vi "mec.vi"() -> ()   [LabVIEW 2016]
uses:
  <instrlib>/ZaberTSeries/Public/Utility/Request.ctl
  <instrlib>/Lake Shore 350/Public/Data/Sensor Data (Single Reading).vi
  <vilib>/Utility/file.llb/Write Delimited Spreadsheet (string).vi
  <vilib>/Utility/file.llb/Write Delimited Spreadsheet (DBL).vi
  <instrlib>/Lake Shore 372/Lake Shore 372.lvlib
  <instrlib>/Lake Shore 350/Lake Shore 350.lvlib
  <instrlib>/Lake Shore Cryotronics 370/Lake Shore Cryotronics 370.lvlib
  <instrlib>/ZaberTSeries/ZaberTSeries.lvlib
panel:
  in  "Stop":bool=TRUE
  out "current time":timestamp format="%<%I:%M:%S %p>T"
  in  "Tab Control":T1(tab)=enum."Ramp Config"
  out "Reading 370":bool
  out "Arduino OK":bool
  out "PT1":waveform(dbl)(graph)
  out "stopping":bool=TRUE
  out "FAA RO600":dbl caption="FAA (K)" min=0.0 max=63200000.0 step=1e-05 format="%_4f"
  out "Sample RuOx":dbl caption="Device (K)" min=0.0 max=63200000.0 step=1e-05 format="%_3f"
  out "Magnet Current (A)":dbl format="%.3f"
  out "77K Diode":dbl format="%_4f"
  out "4K Diode":dbl format="%_4f"
  out "Magnetic Field (kG)":dbl min=-601000.0 max=601000.0 step=0.0001 format="%_3f"
  in  "Auto-Ramp":bool
  in  "ramp start time":timestamp
  out "Ramp Status":string="Shutting down"
  out "Ramp State":u16(ring)=6 items=["Ramp Up", "Soak (hold)", "Ramp Down", "Ramp up to Setpoint", "Closed Loop Feedback", "Ramp down from Setpoint", "Magnet off"]
  out "Magnet Current":waveform(dbl)[](graph)
  out "Device T":waveform(dbl)(graph)
  out "Sample RuOx R":dbl caption="Device R (Ohms)" min=0.0 max=63200000.0 step=1e-05 format="%_3f"
  out "FAA RO600 R":dbl caption="FAA R (Ohms)" min=0.0 max=63200000.0 step=1e-05 format="%_4f"
  out "Magnet RTD":dbl caption="Magnet (K)" format="%.2f"
  out "GGG RO600":dbl caption="GGG (K)" format="%_4f"
  out "GGG RO600 R":dbl caption="GGG R (Ohms)" format="%_4f"
  out "Magnet RTD R":dbl caption="Magnet R (Ohms)" format="%.2f"
  out "PT2":waveform(dbl)(graph)
  in  "magnet control resistance ohms":dbl=20.0
  in  "Calculate Autoramp Time":bool
  in  "End of Ramp Temp Control":bool=TRUE
  in  "soak time (minutes)":dbl=50.0
  out "cycle time (min)":dbl format="%#_3g"
  out "Ramp down step size (mA)":dbl=1.0
  in  "setpoint (K)":dbl=0.09
  in  "Manual temp control":bool
  in  "ls350":refnum<visa-resource-name>="350"
  in  "ls370":refnum<visa-resource-name>="370"
  out "Ramp up step size (%)":dbl=0.02
  out "max magnet value(%)":dbl=10.0
  in  "read lakeshore sensors":bool=TRUE
  in  "Record Temps":bool=TRUE
  in  "Timeout (ms)":i32=2000
  out "Ramp up step size (mA)":dbl=1.0
  in  "Max current (A)":dbl=9.4
  in  "thermo data path":path=path "C:/data/temperature_log/mec"
  in  "Field constant (kG/A)":dbl=4.566 min=0.001 max=10.0 step=1e-05 format="%.3f"
  out "Ramp down step size (%)":dbl=0.02
  out "ramp up time (min)":dbl=60.0
  out "ramp down time (min)":dbl=60.0
  out "ramp down start time":timestamp
  in  "Ramp up rate (mA/s)":dbl=5.0
  in  "Ramp down rate (mA/s)":dbl=5.0
  in  "Heat Switch":bool
  in  "Ramp Magnet Up":bool
  in  "Ramp Magnet Down":bool
  in  "control channel":string="1"
  out "counter":dbl
  in  "delay after ramp down (min)":dbl=20.0
  out "counter 2":dbl
  out "ramp finish time":timestamp
  out "lakeshore output %":dbl format="%.3f"
  out "Heater Range Set":u16(ring) items=["Off", "31.6 uA", "100 uA", "316 uA", "1.00 mA", "3.16 mA", "10.0 mA", "31.6 mA", "100 mA"]
  out "Heater Range Actual":u16(ring) items=["Off", "31.6 uA", "100 uA", "316 uA", "1.00 mA", "3.16 mA", "10.0 mA", "31.6 mA", "100 mA"]
  out "Magnet resistance ohms":dbl=1.0
  out "Heater Range OK":bool
  out "heater Setpoint":dbl min=0.0 max=100000000.0 step=1e-06 format="%.5f"
  out "lakeshore output current mA":dbl
  out "kepco input voltage (V)":dbl
  out "kepco output voltage (V)":dbl
  out "Magnet Current (A) 2":dbl format="%.3f"
  in  "magnet ramp resistance ohms":dbl=0.1005
  in  "Update PID Values":bool
  in  "Warmup Heater":bool=TRUE
  in  "Channel (1)":u16(ring)=1 items=["1"=1, "2"=2, "3"=3, "4"=4, "5"=5, "6"=6, "7"=7, "8"=8, "9"=9, "10"=10, "11"=11, "12"=12, "13"=13, "14"=14, "15"=15, "16"=16, "A (Control Input)"=17]
  in  "Excitation Range (5: 200 uV / 100 pA)":u16(ring)=5 items=["2.00 uV / 1.00 pA"=1, "6.32 uV / 3.16 pA"=2, "20.0 uV / 10.0 pA"=3, "63.2 uV / 31.6 pA"=4, "200 uV / 100 pA"=5, "632 uV / 316 pA"=6, "2.00 mV / 1.00 nA"=7, "6.32 mV / 3.16 nA"=8, "20.0 mV / 10.0 nA"=9, "63.2 mV / 31.6 nA"=10, "200 mV / 100 nA"=11, "632 mV / 316 nA"=12, "1.00 uA"=13, "3.16 uA"=14, "10.0 uA"=15, "31.6 uA"=16, "100 uA"=17, "316 uA"=18, "1.00 mA"=19, "3.16 mA"=20, "10.0 mA"=21, "31.6 mA"=22]
  in  "Autorange (0: Autorange off)":u16(ring) items=["Autorange off", "Autorange Current", "ROX 102B Autorange"]
  in  "Excitation  (T: On)":bool=TRUE
  in  "Excitation Mode (0: Voltage)":u16(ring) items=["Voltage", "Current"]
  in  "Resistance Range (17: 200 kOhm)":u16(ring)=17 items=["2.00 mOhm"=1, "6.32 mOhm"=2, "20.0 mOhm"=3, "63.2 mOhm"=4, "200 mOhm"=5, "632 mOhm"=6, "2.00 Ohm"=7, "6.32 Ohm"=8, "20.0 Ohm"=9, "63.2 Ohm"=10, "200 Ohm"=11, "632 Ohm"=12, "2.00 kOhm"=13, "6.32 kOhm"=14, "20.0 kOhm"=15, "63.2 kOhm"=16, "200 kOhm"=17, "632 kOhm"=18, "2.00 MOhm"=19, "6.32 MOhm"=20, "20.0 MOhm"=21, "63.2 MOhm"=22]
  in  "Gain(P)":dbl=1.1 min=0.001 max=1000.0 step=0.001 format="%.3f"
  in  "Reset(I)":dbl=30.0 min=0.0 max=10000.0 step=1.0
  in  "Rate(D)":dbl min=0.0 max=2500.0 step=1.0
  in  "Mode (0:Off)":u16(ring)=3 items=["Off", "Closed Loop PID", "Zone", "Open Loop"]
  in  "Heater Output (1:1)":u16(ring)=1 items=["1"=1, "2"=2]
  in  "Input (0:None)":u16(ring)=6 items=["None", "A", "B", "C", "D", "D2", "D3", "D4", "D5"]
  in  "Max Current (0:User Specified)":u16(ring) items=["User Specified", "0.707 A", "1.0 A", "1.141 A", "2.0 A"]
  in  "Heater Out Display (1:Current)":u16(ring)=1 items=["Current"=1, "Power"=2]
  in  "Max User Current (2.000)":dbl=0.1 format="%.3f"
  in  "Heater Resistance (1:25 Ohms)":u16(ring)=2 items=["25 Ohms"=1, "50 Ohms"=2]
  in  "heater output":u16(ring)=1 items=["1"=1, "2"=2, "3"=3, "4"=4]
  in  "warmup heater Range":u16(ring) items=["Off", "Range 1 (On)", "Range 2", "Range 3", "Range 4", "Range 5"]
  in  "warmup heater output %":dbl=62.0 format="%.2f"
  in  "Knob":i8(knob) scale=0.0..2.0
  in  "auto-read HEMT voltages":bool=TRUE
  in  "Read ADC current":bool=TRUE
  in  "query adc magnet current once":bool
  in  "MUX relays":bool
  in  "Query all HEMT voltages once":bool
  out "HEMT biases":dbl[][](array[numeric])
  out "ADC0 outputs":dbl[][](array[numeric])
  out "adc magnet current (A)":dbl
  in  "Arduino":refnum<visa-resource-name>="COM6"
  out "flow meter":dbl
  out "hemt v counter":i32
  out "element":string
  out "last record time":dbl
  in  "HEMT data path":path=path "C:/data/temperature_log/mec"
  out "error out":errorcluster
  out "Flow Meter":waveform(dbl)(graph)
  out "FAA T":waveform(dbl)(graph)={"t0"=timestamp(3512160360.4800687 s since 1904-01-01), "dt"=0.0, "Y"=[0.0]}
  out "GGG T":waveform(dbl)(graph)={"t0"=timestamp(3512160360.4800687 s since 1904-01-01), "dt"=0.0, "Y"=[0.0]}
  out "magnet RTD R":waveform(dbl)(graph)={"t0"=timestamp(3512160360.4800687 s since 1904-01-01), "dt"=0.0, "Y"=[0.0]}
  in  "initialize":bool
  # "MEC!"
  # "ADR CONTROL"
  # "Manual ADR CONTROL"
  # "How often to measure temps?\nDon't change this during ramps."
  # "OPEN"
  # "CLOSED"
  # "Ramp Parameters"
  # "\"A\" for Darkness \n\"1\" for MEC"
  # "Lakeshore 370"
  # "Warmup Heater (LS350)"
  # "Temp Control Parameters\nLS370"
  # "ON"
  # "OFF"
  # "ARCONS used 1.1, 60, and 15 for PID"
  # "A1"
  # "A2"
  # "A3"
  # "OFF"
  # "ON"
  # "A4"
  # "A5"
  # "B1"
  # "OPEN"
  # "CLOSED"
  # "B2"
  # "last HEMT voltage polled:"
  # "B3"
  # "B4"
  # "B5"
  # "Vd (mV)"
  # "Id (mAx100)"
  # "Vg (mV)"
  # "magnet \ncurrent"
  # "flow \nmeter"
  # "OFF"
  # "ON"
  # "Thermometers\n\nFrom DARKNESS\nUse ~ 20 uV or ~20 nA excitation for FAA and device thermometers. \nHPD recommendations (these are conservative. Scientific instruments used excitations that were 10 to 100 times higher)\nT(K)                            excitation (nA)\n.175 to 4.2                  10\n.1 to .175                    3\n<.1                              0.1\n\nDiodes get 10 uA excitation. \n\n\nKepco Front Panel\nVoltage Control = OFF\nCurrent Control = OFF\nMode = Voltage\n\nSample Heater Output from LS372 connects to Voltage Programming Input on Kepco. Red terminal on front of Kepco should\nget a voltage <0, Red magnet wire goes to OUT on back of Kepco, Blue wire goes to COM on back of Kepco."
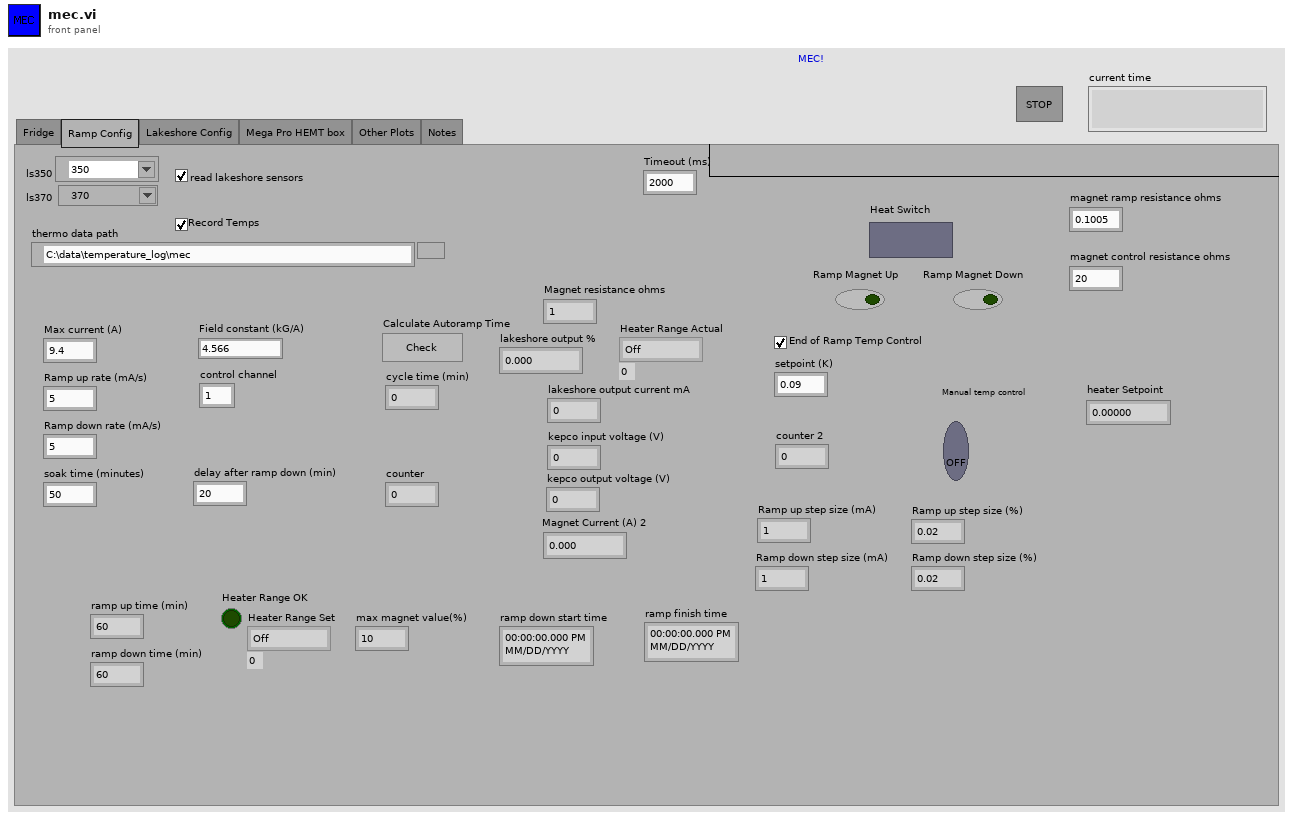
[diagram p1: front panel]
types:
  T1 = enum32{"Fridge", "Ramp Config", "Lakeshore Config", "Mega Pro HEMT box", "Other Plots", "Notes"}
  T2 = typedef "ZaberTSeries.lvlib/Request.ctl" = cluster{"Device Number":u8, "Command":u8, "Data":i32, "Response Count":i32}
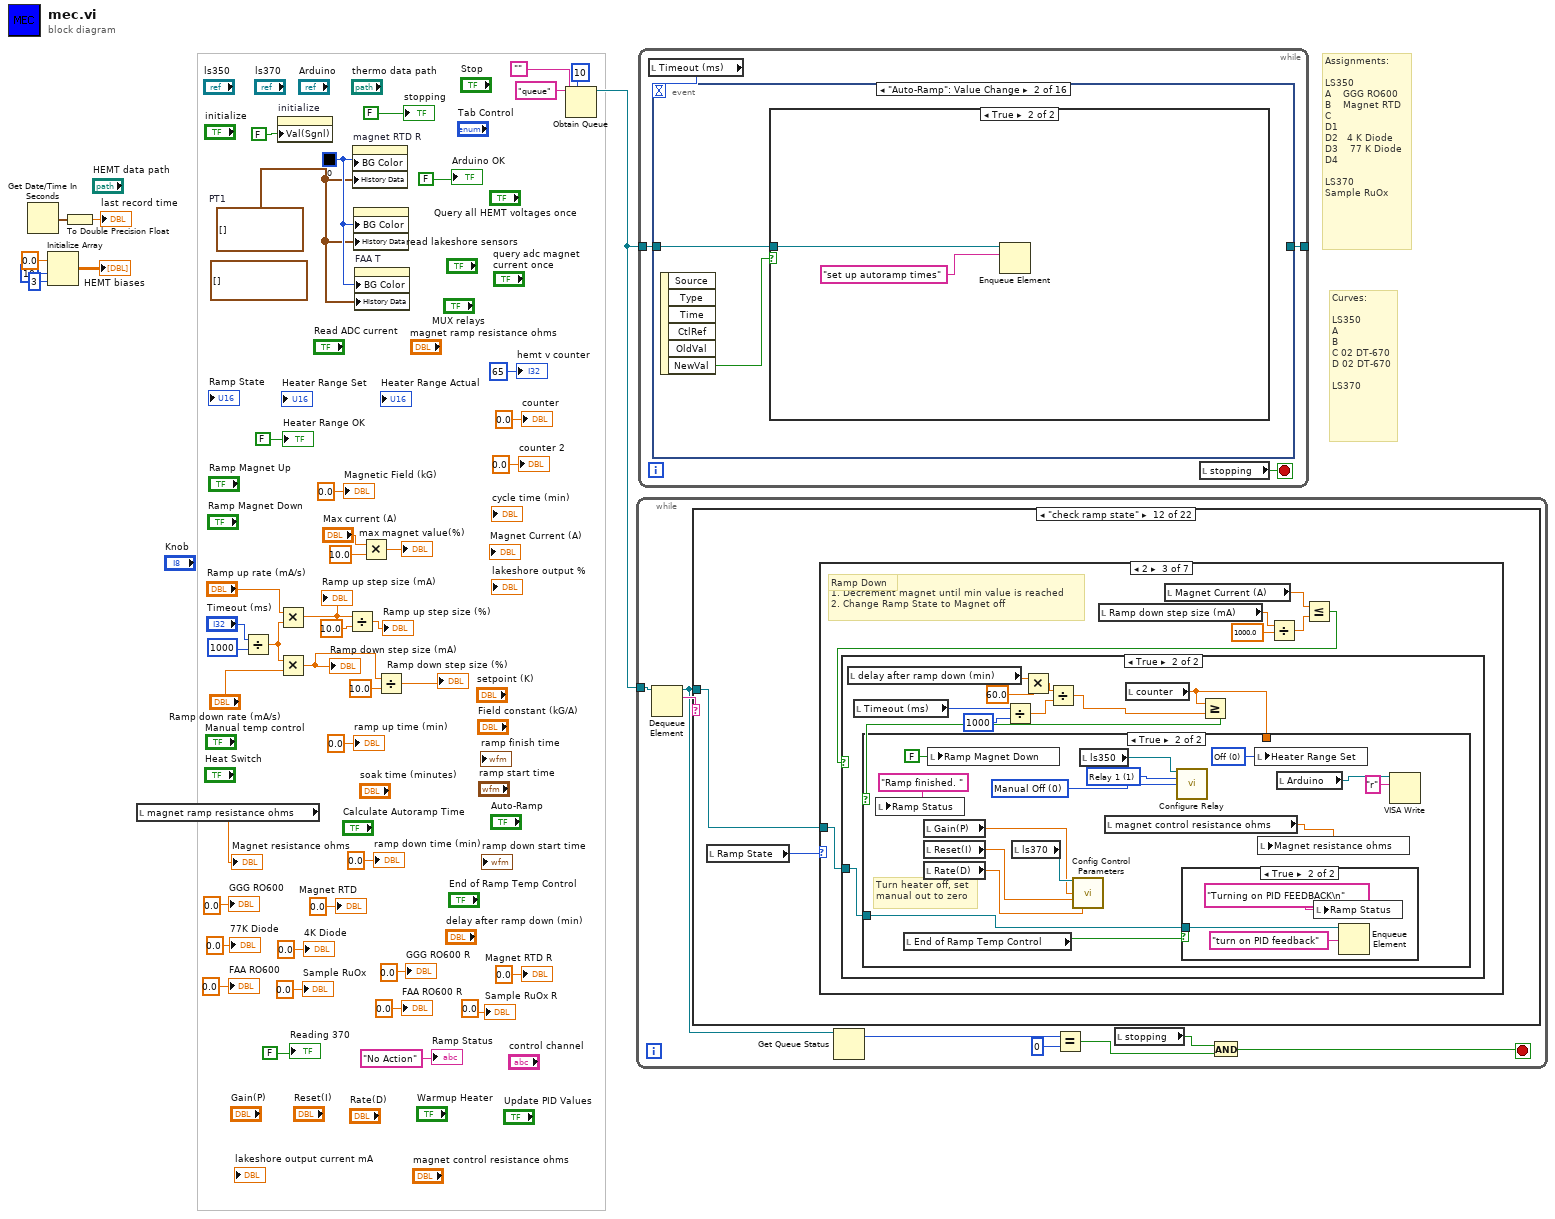
[diagram p0: block diagram]
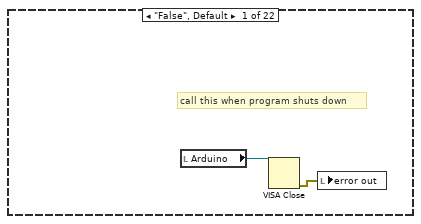
[diagram p2: hidden frame]
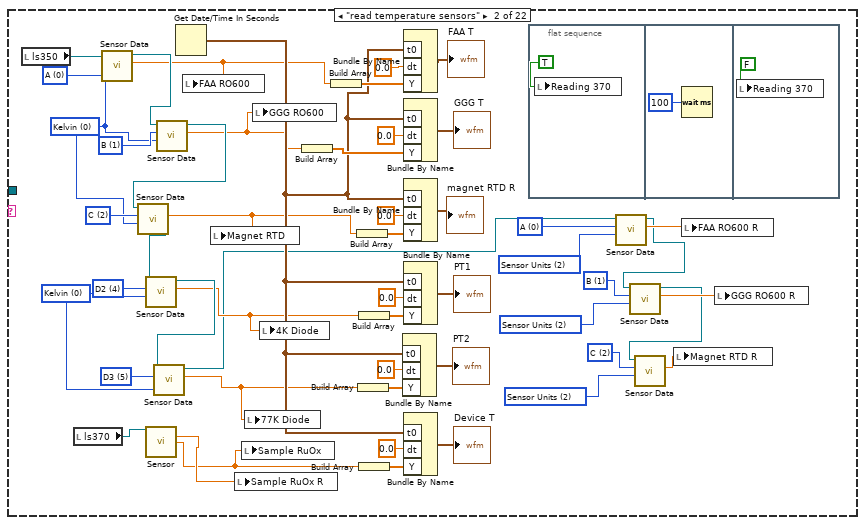
[diagram p3: hidden frame]
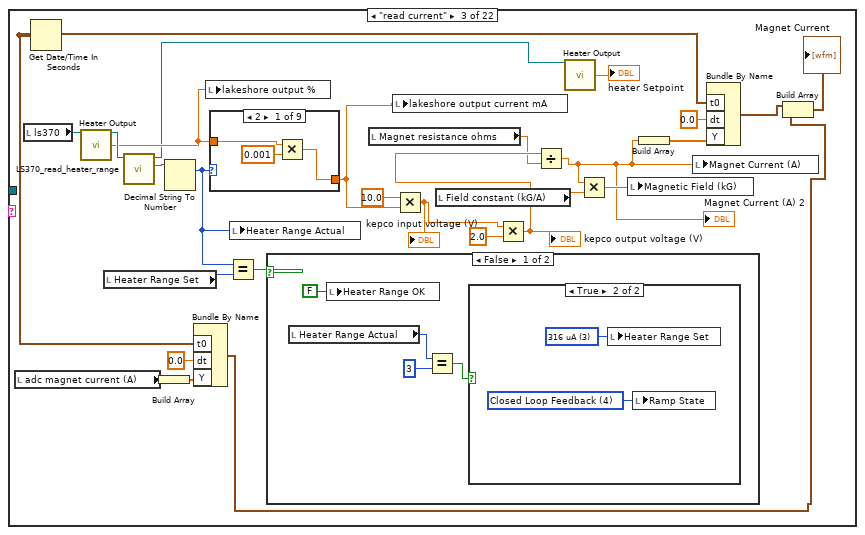
[diagram p4: hidden frame]
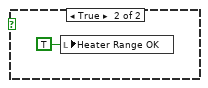
[diagram p6: hidden frame]
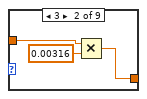
[diagram p7: hidden frame]
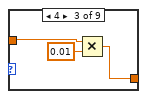
[diagram p8: hidden frame]
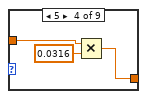
[diagram p9: hidden frame]
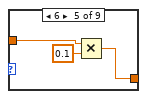
[diagram p10: hidden frame]
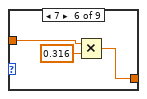
[diagram p11: hidden frame]
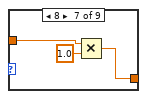
[diagram p12: hidden frame]
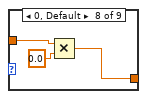
[diagram p13: hidden frame]
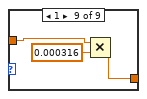
[diagram p14: hidden frame]
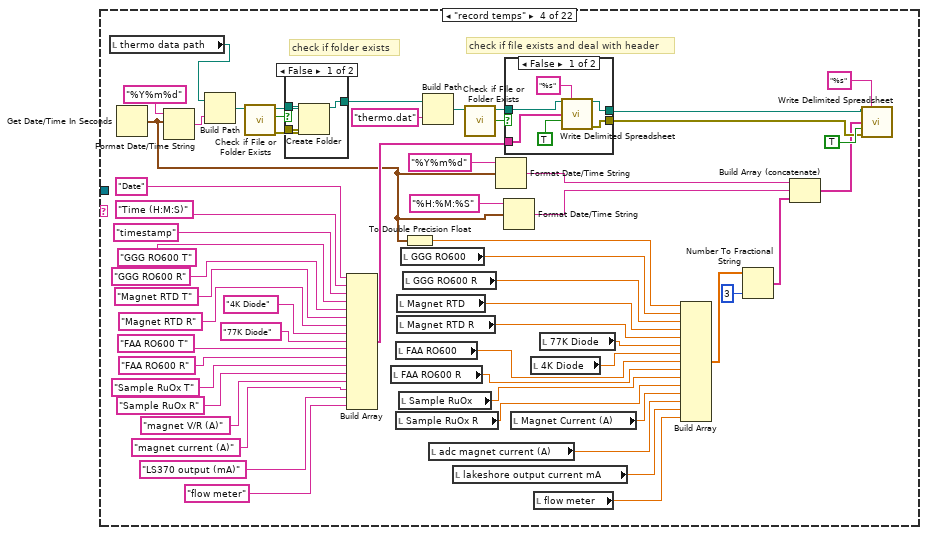
[diagram p15: hidden frame]
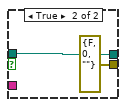
[diagram p16: hidden frame]
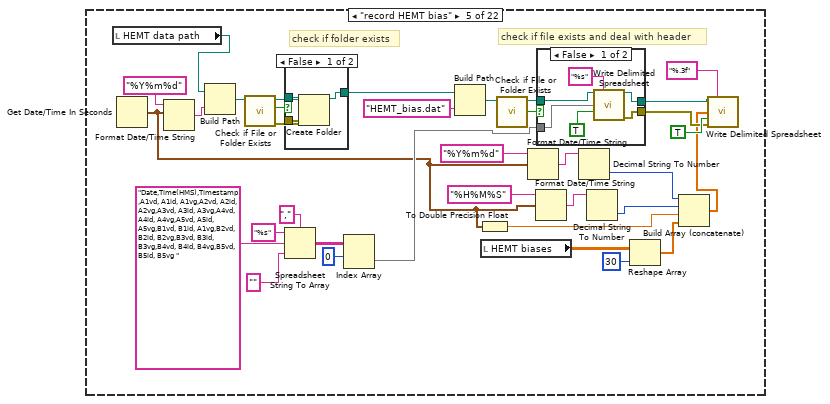
[diagram p18: hidden frame]
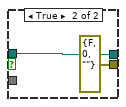
[diagram p19: hidden frame]
diagram:
  (unwired) waveform(dbl)[][] [] ("History Data")
  w9 = waveform(dbl)[] [] ("History Data")
  w39 = u32 0
  # "Curves:\n\nLS350\nA\nB\nC 02 DT-670\nD 02 DT-670\n\nLS370"
  # "Assignments:\n\nLS350\nA    GGG RO600 \nB    Magnet RTD\nC\nD1\nD2   4 K Diode\nD3    77 K Diode\nD4\n\nLS370\nSample RuOx"
  n1 = Get Date/Time In Seconds() -> (seconds since 1Jan1904=w6:timestamp)
  n2 = Initialize Array(0.0 ("element"), 10 ("dimension size"), 3 ("dimension size")) -> (→"HEMT biases":dbl[][])
  n3 = To Double Precision Float(number=w6) -> (double precision float=→"last record time":dbl)
  n4 = local read "magnet ramp resistance ohms"() -> (→"Magnet resistance ohms":dbl)
  n5 = Divide(x="Timeout (ms)", y=1000) -> (x/y=w19:dbl)
  n6 = property on="initialize" class="Bool (strict)"("Val(Sgnl)"=FALSE ("Boolean")) -> ()  [unwired: 2 in, 2 out]
  n7 = Multiply(x="Ramp up rate (mA/s)", y=w19) -> (x*y=w16:dbl)
  "Ramp up step size (mA)" <- w16
  n8 = Multiply(x=w19, y="Ramp down rate (mA/s)") -> (x*y=w17:dbl)
  "Ramp down step size (mA)" <- w17
  n9 = Divide(x=w16, y=10.0) -> (x/y=→"Ramp up step size (%)":dbl)
  n10 = property on="magnet RTD R" class="WFChart (strict)"("BG Color"=w39, "History Data"=w9) -> ()  [unwired: 2 in, 2 out]
  n11 = property on="PT1" class="WFChart (strict)"("BG Color"=w39, "History Data"=w9) -> ()  [unwired: 2 in, 2 out]
  n12 = property on="FAA T" class="WFChart (strict)"("BG Color"=w39, "History Data"=w9) -> ()  [unwired: 2 in, 2 out]
  n13 = Multiply(x="Max current (A)", y=10.0) -> (x*y=→"max magnet value(%)":dbl)
  n14 = Divide(x=w17, y=10.0) -> (x/y=→"Ramp down step size (%)":dbl)
  n15 = Obtain Queue(max queue size (-1, unlimited)=10, name (unnamed)="queue", element data type="") -> (queue out=w47:refnum<queue>)  [unwired: 2 in, 2 out]
  n16 = while {
    tunnel: w47 -> [w57]
    stop <- w51 stop-if-true
    n17 = Dequeue Element(queue=w57) -> (queue out=w50:refnum<queue>, element=w56:string)  [unwired: 2 in, 2 out]
    n18 = case shown="\"check ramp state\"" w56 {
      tunnel: w50 -> [_ _ _ _ _ _ _ _ _ _ _ w489 _ _ _ _ _ _ _ _ _ _]
      frame "False", Default {
        # "call this when program shuts down"
        n19 = local read "Arduino"() -> (w59:refnum<visa-resource-name>)
        n20 = VISA Close(VISA resource name=w59) -> (error out=w58:errorcluster)  [unwired: 1 in]
        n21 = local write "error out"(w58) -> ()
      }
      frame "read temperature sensors" {
        w61 = u16 2 items=["Kelvin", "Celsius", "Sensor Units"] ("Data Source (0:Kelvin)")
        w63 = u16 2 items=["A", "B", "C", "D", "D2", "D3", "D4", "D5"] ("Input (0:A)")
        w67 = u16 2 items=["Kelvin", "Celsius", "Sensor Units"] ("Data Source (0:Kelvin)")
        w65 = u16 1 items=["A", "B", "C", "D", "D2", "D3", "D4", "D5"] ("Input (0:A)")
        w70 = u16 2 items=["Kelvin", "Celsius", "Sensor Units"] ("Data Source (0:Kelvin)")
        w71 = u16 0 items=["A", "B", "C", "D", "D2", "D3", "D4", "D5"] ("Input (0:A)")
        w94 = u16 5 items=["A", "B", "C", "D", "D2", "D3", "D4", "D5"] ("Input (0:A)")
        w92 = u16 0 items=["Kelvin", "Celsius", "Sensor Units"] ("Data Source (0:Kelvin)")
        w95 = u16 4 items=["A", "B", "C", "D", "D2", "D3", "D4", "D5"] ("Input (0:A)")
        w99 = u16 2 items=["A", "B", "C", "D", "D2", "D3", "D4", "D5"] ("Input (0:A)")
        w97 = u16 0 items=["Kelvin", "Celsius", "Sensor Units"] ("Data Source (0:Kelvin)")
        w100 = u16 1 items=["A", "B", "C", "D", "D2", "D3", "D4", "D5"] ("Input (0:A)")
        w104 = u16 0 items=["A", "B", "C", "D", "D2", "D3", "D4", "D5"] ("Input (0:A)")
        n22 = local read "ls350"() -> (w105:refnum<visa-resource-name>)
        n23 = local read "ls370"() -> (w83:refnum<visa-resource-name>)
        n24 = call-poly <instrlib>:"Sensor Data.vi"("Data Source (0:Kelvin)"=w97, "Input (0:A)"=w104, "VISA resource name"=w105) -> ("Sensor Data"=w78:dbl, "VISA resource name out"=w101:refnum<visa-resource-name>)  [unwired: 6 in, 1 out]
        n25 = call <instrlib>:"Sensor.vi"("VISA resource name"=w83) -> ("Resistance Reading"=w74:dbl, "Kelvin Reading"=w73:dbl)  [unwired: 10 in, 3 out]
        n26 = call-poly <instrlib>:"Sensor Data.vi"("Data Source (0:Kelvin)"=w97, "Input (0:A)"=w100, "VISA resource name"=w101) -> ("Sensor Data"=w69:dbl, "VISA resource name out"=w98:refnum<visa-resource-name>)  [unwired: 6 in, 1 out]
        n27 = call-poly <instrlib>:"Sensor Data.vi"("Data Source (0:Kelvin)"=w97, "Input (0:A)"=w99, "VISA resource name"=w98) -> ("Sensor Data"=w77:dbl, "VISA resource name out"=w96:refnum<visa-resource-name>)  [unwired: 6 in, 1 out]
        n28 = call-poly <instrlib>:"Sensor Data.vi"("Data Source (0:Kelvin)"=w92, "Input (0:A)"=w95, "VISA resource name"=w96) -> ("Sensor Data"=w75:dbl, "VISA resource name out"=w93:refnum<visa-resource-name>)  [unwired: 6 in, 1 out]
        n29 = call-poly <instrlib>:"Sensor Data.vi"("Data Source (0:Kelvin)"=w92, "Input (0:A)"=w94, "VISA resource name"=w93) -> ("Sensor Data"=w76:dbl, "VISA resource name out"=w72:refnum<visa-resource-name>)  [unwired: 6 in, 1 out]
        n30 = Get Date/Time In Seconds() -> (seconds since 1Jan1904=w79:timestamp)
        n31 = local write "FAA RO600"(w78) -> ()
        n32 = local write "Magnet RTD"(w77) -> ()
        n33 = local write "Sample RuOx R"(w74) -> ()
        n34 = local write "Sample RuOx"(w73) -> ()
        n35 = local write "77K Diode"(w76) -> ()
        n36 = local write "GGG RO600"(w69) -> ()
        n37 = local write "4K Diode"(w75) -> ()
        n38 = Build Array(w69) -> (w90:dbl[])
        n39 = Build Array(w78) -> (w102:dbl[])
        n40 = Build Array(w77) -> (w89:dbl[])
        n41 = Build Array(w76) -> (w84:dbl[])
        n42 = Build Array(w75) -> (w87:dbl[])
        n43 = Build Array(w73) -> (w82:dbl[])
        n44 = Bundle By Name("t0"=w79, "dt"=0.0, "Y"=w84) -> (→"PT2":waveform(dbl))  [unwired: 1 in]
        n45 = Bundle By Name("t0"=w79, "dt"=0.0, "Y"=w102) -> (→"FAA T":waveform(dbl))  [unwired: 1 in]
        n46 = Bundle By Name("t0"=w79, "dt"=0.0, "Y"=w90) -> (→"GGG T":waveform(dbl))  [unwired: 1 in]
        n47 = Bundle By Name("t0"=w79, "dt"=0.0, "Y"=w89) -> (→"magnet RTD R":waveform(dbl))  [unwired: 1 in]
        n48 = Bundle By Name("t0"=w79, "dt"=0.0, "Y"=w87) -> (→"PT1":waveform(dbl))  [unwired: 1 in]
        n49 = Bundle By Name("t0"=w79, "dt"=0.0, "Y"=w82) -> (→"Device T":waveform(dbl))  [unwired: 1 in]
        n50 = flat-sequence {
          frame #0 {
            n51 = local write "Reading 370"(TRUE ("Reading 370")) -> ()
          }
          frame #1 {
            n52 = Wait (ms)(milliseconds to wait=u32 100) -> ()  [unwired: 1 out]
          }
          frame #2 {
            n53 = local write "Reading 370"(FALSE ("Reading 370")) -> ()
          }
        }
        n54 = call-poly <instrlib>:"Sensor Data.vi"("Data Source (0:Kelvin)"=w70, "Input (0:A)"=w71, "VISA resource name"=w72) -> ("Sensor Data"=w68:dbl, "VISA resource name out"=w64:refnum<visa-resource-name>)  [unwired: 6 in, 1 out]
        n55 = call-poly <instrlib>:"Sensor Data.vi"("Data Source (0:Kelvin)"=w67, "Input (0:A)"=w65, "VISA resource name"=w64) -> ("Sensor Data"=w66:dbl, "VISA resource name out"=w60:refnum<visa-resource-name>)  [unwired: 6 in, 1 out]
        n56 = call-poly <instrlib>:"Sensor Data.vi"("Data Source (0:Kelvin)"=w61, "Input (0:A)"=w63, "VISA resource name"=w60) -> ("Sensor Data"=w62:dbl)  [unwired: 6 in, 2 out]
        n57 = local write "Magnet RTD R"(w62) -> ()
        n58 = local write "FAA RO600 R"(w68) -> ()
        n59 = local write "GGG RO600 R"(w66) -> ()
      }
      frame "read current" {
        n60 = local read "adc magnet current (A)"() -> (w119:dbl)
        n61 = local read "ls370"() -> (w138:refnum<visa-resource-name>)
        n62 = Get Date/Time In Seconds() -> (seconds since 1Jan1904=w115:timestamp)
        n63 = call <instrlib>:"Heater Output.vi"("VISA resource name"=w138) -> ("VISA resource name out"=w137:refnum<visa-resource-name>, "Heater Output"=w132:dbl)  [unwired: 12 in, 1 out]
        n64 = local read "Heater Range Set"() -> (w134:u16)
        n65 = call "LS370_read_heater_range.vi"("VISA resource name"=w137) -> ("heater range"=w136:string, "VISA resource name out"=w129:refnum<visa-resource-name>)  [unwired: 9 in]
        n66 = Build Array(w119) -> (w120:dbl[])
        n67 = Decimal String To Number(string=w136) -> (number=w135:i32)  [unwired: 2 in, 1 out]
        n68 = Bundle By Name("t0"=w115, "dt"=0.0, "Y"=w120) -> (w117:waveform(dbl))  [unwired: 1 in]
        n69 = local write "lakeshore output %"(w132) -> ()
        n70 = case shown="2" w135 {
          tunnel: [w148 w151 w154 w157 w160 w163 w166 w169 w173] -> w114
          tunnel: w132 -> [w149 w152 w155 w158 w161 w164 w167 w170 w172]
          frame 2 {
            n71 = Multiply(x=w149, y=0.001) -> (x*y=w148:dbl)
          }
          frame 3 {
            n72 = Multiply(x=w152, y=0.00316) -> (x*y=w151:dbl)
          }
          frame 4 {
            n73 = Multiply(x=w155, y=0.01) -> (x*y=w154:dbl)
          }
          frame 5 {
            n74 = Multiply(x=w158, y=0.0316) -> (x*y=w157:dbl)
          }
          frame 6 {
            n75 = Multiply(x=w161, y=0.1) -> (x*y=w160:dbl)
          }
          frame 7 {
            n76 = Multiply(x=w164, y=0.316) -> (x*y=w163:dbl)
          }
          frame 8 {
            n77 = Multiply(x=w167, y=1.0) -> (x*y=w166:dbl)
          }
          frame 0, Default {
            n78 = Multiply(x=w170, y=0.0) -> (x*y=w169:dbl)
          }
          frame 1 {
            n79 = Multiply(x=w172, y=0.000316) -> (x*y=w173:dbl)
          }
        }
        n80 = Equal?(x=w135, y=w134) -> (x = y?=w133:bool)
        n81 = local write "Heater Range Actual"(w135) -> ()
        n82 = case shown="False" w133 {
          frame False {
            n83 = local read "Heater Range Actual"() -> (w141:u16)
            n84 = local write "Heater Range OK"(FALSE ("Heater Range OK")) -> ()
            n85 = Equal?(x=w141, y=u16 3) -> (x = y?=w143:bool)
            n86 = case shown="True" w143 {
              frame False {
              }
              frame True {
                w145 = u16 3 items=["Off", "31.6 uA", "100 uA", "316 uA", "1.00 mA", "3.16 mA", "10.0 mA", "31.6 mA", "100 mA"] ("Heater Range Set")
                w146 = u16 4 items=["Ramp Up", "Soak (hold)", "Ramp Down", "Ramp up to Setpoint", "Closed Loop Feedback", "Ramp down from Setpoint", "Magnet off"] ("Ramp State")
                n87 = local write "Heater Range Set"(w145) -> ()
                n88 = local write "Ramp State"(w146) -> ()
              }
            }
          }
          frame True {
            n89 = local write "Heater Range OK"(TRUE ("Heater Range OK")) -> ()
          }
        }
        n90 = local read "Magnet resistance ohms"() -> (w123:dbl)
        n91 = local write "lakeshore output current mA"(w114) -> ()
        n92 = Multiply(x=10.0, y=w114) -> (x*y=w126:dbl)
        "kepco input voltage (V)" <- w126
        n93 = local read "Field constant (kG/A)"() -> (w140:dbl)
        n94 = Multiply(x=w126, y=2.0) -> (x*y=w124:dbl)
        "kepco output voltage (V)" <- w124
        n95 = Divide(x=w124, y=w123) -> (x/y=w122:dbl)
        "Magnet Current (A) 2" <- w122
        n96 = call <instrlib>:"Heater Output.vi"("VISA resource name"=w129) -> ("Heater Output"=→"heater Setpoint":dbl)  [unwired: 12 in, 2 out]
        n97 = Multiply(x=w122, y=w140) -> (x*y=w139:dbl)
        n98 = local write "Magnetic Field (kG)"(w139) -> ()
        n99 = Build Array(w122) -> (w131:dbl[])
        n100 = local write "Magnet Current (A)"(w122) -> ()
        n101 = Bundle By Name("t0"=w115, "dt"=0.0, "Y"=w131) -> (w118:waveform(dbl))  [unwired: 1 in]
        n102 = Build Array(w118, w117) -> (→"Magnet Current":waveform(dbl)[])
      }
      frame "record temps" {
        # "check if file exists and deal with header"
        # "check if folder exists"
        n103 = local read "thermo data path"() -> (w196:path)
        n104 = Get Date/Time In Seconds() -> (seconds since 1Jan1904=w189:timestamp)
        n105 = Format Date/Time String(time format string (%c)="%Y%m%d", seconds (now)=w189) -> (date/time string=w222:string)  [unwired: 1 in]
        n106 = Build Path(base path=w196, name or relative path=w222) -> (appended path=w224:path)
        n107 = call <vilib>:"Check if File or Folder Exists.vi"("path"=w224) -> ("error out"=w227:errorcluster, "file or folder exists?"=w226:bool, "dup path"=w225:path)  [unwired: 8 in]
        n108 = case shown="False" w226 {
          tunnel: w225 -> [w243 w244]
          tunnel: w227 -> [w242 _]
          tunnel: [w241 w244] -> w228
          frame False {
            n109 = Create Folder(path (use dialog)=w243, error in=w242) -> (created path=w241:path)  [unwired: 1 in, 2 out]
          }
          frame True {
          }
        }
        n110 = Build Array("Date" ("element"), "Time (H:M:S)" ("element"), "timestamp" ("element"), "GGG RO600 T" ("element"), "GGG RO600 R" ("element"), "Magnet RTD T" ("element"), "Magnet RTD R" ("element"), "4K Diode" ("element"), "77K Diode" ("element"), "FAA RO600 T" ("element"), "FAA RO600 R" ("element"), "Sample RuOx T" ("element"), "Sample RuOx R" ("element"), "magnet V/R (A)" ("element"), "magnet current (A)" ("element"), "LS370 output (mA)" ("element"), "flow meter" ("element")) -> (w219:string[])
        n111 = local read "FAA RO600 R"() -> (w199:dbl)
        n112 = local read "FAA RO600"() -> (w200:dbl)
        n113 = local read "Sample RuOx R"() -> (w197:dbl)
        n114 = local read "Magnet RTD"() -> (w204:dbl)
        n115 = local read "Magnet RTD R"() -> (w203:dbl)
        n116 = local read "Sample RuOx"() -> (w198:dbl)
        n117 = local read "GGG RO600"() -> (w232:dbl)
        n118 = local read "GGG RO600 R"() -> (w205:dbl)
        n119 = To Double Precision Float(number=w189) -> (double precision float=w217:dbl)
        n120 = Build Path(base path=w228, name or relative path="thermo.dat") -> (appended path=w229:path)
        n121 = local read "adc magnet current (A)"() -> (w183:dbl)
        n122 = local read "lakeshore output current mA"() -> (w184:dbl)
        n123 = call <vilib>:"Check if File or Folder Exists.vi"("path"=w229) -> ("file or folder exists?"=w230:bool, "dup path"=w231:path)  [unwired: 8 in, 1 out]
        n124 = Format Date/Time String(time format string (%c)="%Y%m%d", seconds (now)=w189) -> (date/time string=w180:string)  [unwired: 1 in]
        n125 = Format Date/Time String(time format string (%c)="%H:%M:%S", seconds (now)=w189) -> (date/time string=w179:string)  [unwired: 1 in]
        n126 = case shown="False" w230 {
          tunnel: [w234 w240] -> w195
          tunnel: w231 -> [w237 w240]
          tunnel: w219 -> [w236 _]
          tunnel: [w233 errorcluster {"status"=FALSE, "code"=0, "source"=""} ("error out")] -> w182
          frame False {
            n127 = call-poly <vilib>:"Write Delimited Spreadsheet.vi"("file path (dialog if empty)"=w237, "format (%s)"="%s" ("format (%.3f)"), "1D data"=w236, "append to file? (new file:F)"=TRUE) -> ("new file path (Not A Path if cancelled)"=w234:path, "error out"=w233:errorcluster)  [unwired: 10 in]
          }
          frame True {
          }
        }
        n128 = local read "Magnet Current (A)"() -> (w206:dbl)
        n129 = local read "4K Diode"() -> (w201:dbl)
        n130 = local read "flow meter"() -> (w185:dbl)
        n131 = local read "77K Diode"() -> (w202:dbl)
        n132 = Build Array(w217, w232, w205, w204, w203, w202, w201, w200, w199, w198, w197, w206, w183, w184, w185) -> (w177:dbl[])
        n133 = Number To Fractional String(number=w177, precision (6)=i16 3) -> (F-format string=w176:string[])  [unwired: 2 in]
        n134 = Build Array (concatenate)(w180, w179, w176) -> (w175:string[])
        n135 = call-poly <vilib>:"Write Delimited Spreadsheet.vi"("file path (dialog if empty)"=w195, "format (%s)"="%s" ("format (%.3f)"), "1D data"=w175, "append to file? (new file:F)"=TRUE, "error in (no error)"=w182) -> ()  [unwired: 9 in, 2 out]
      }
      frame "record HEMT bias" {
        # "check if file exists and deal with header"
        # "check if folder exists"
        n136 = local read "HEMT data path"() -> (w268:path)
        n137 = Get Date/Time In Seconds() -> (seconds since 1Jan1904=w246:timestamp)
        n138 = Format Date/Time String(time format string (%c)="%Y%m%d", seconds (now)=w246) -> (date/time string=w270:string)  [unwired: 1 in]
        n139 = Build Path(base path=w268, name or relative path=w270) -> (appended path=w272:path)
        n140 = call <vilib>:"Check if File or Folder Exists.vi"("path"=w272) -> ("error out"=w275:errorcluster, "file or folder exists?"=w274:bool, "dup path"=w273:path)  [unwired: 8 in]
        n141 = case shown="False" w274 {
          tunnel: w273 -> [w290 w291]
          tunnel: w275 -> [w289 _]
          tunnel: [w288 w291] -> w276
          frame False {
            n142 = Create Folder(path (use dialog)=w290, error in=w289) -> (created path=w288:path)  [unwired: 1 in, 2 out]
          }
          frame True {
          }
        }
        n143 = Spreadsheet String To Array(delimiter (Tab)=",", format string="%s", spreadsheet string="Date,Time(HMS),Timestamp,A1vd, A1id, A1vg,A2vd, A2id, A2vg,A3vd, A3id, A3vg,A4vd, A4id, A4vg,A5vd, A5id, A5vg,B1vd, B1id, A1vg,B2vd, B2id, B2vg,B3vd, B3id, B3vg,B4vd, B4id, B4vg,B5vd, B5id, B5vg ", array type (2D Dbl)="") -> (array=w255:string[][])
        n144 = Index Array(array=w255, index (row)=0) -> (element=w253:string[])  [unwired: 1 in]
        n145 = Build Path(base path=w276, name or relative path="HEMT_bias.dat") -> (appended path=w277:path)
        n146 = To Double Precision Float(number=w246) -> (double precision float=w247:dbl)
        n147 = local read "HEMT biases"() -> (w252:dbl[][])
        n148 = call <vilib>:"Check if File or Folder Exists.vi"("path"=w277) -> ("file or folder exists?"=w278:bool, "dup path"=w279:path)  [unwired: 8 in, 1 out]
        n149 = Format Date/Time String(time format string (%c)="%Y%m%d", seconds (now)=w246) -> (date/time string=w264:string)  [unwired: 1 in]
        n150 = Format Date/Time String(time format string (%c)="%H%M%S", seconds (now)=w246) -> (date/time string=w263:string)  [unwired: 1 in]
        n151 = case shown="False" w278 {
          tunnel: [w282 w287] -> w267
          tunnel: w279 -> [w284 w287]
          tunnel: [w281 errorcluster {"status"=FALSE, "code"=0, "source"=""} ("error out")] -> w261
          tunnel: w253 -> [w280 _]
          frame False {
            n152 = call-poly <vilib>:"Write Delimited Spreadsheet.vi"("file path (dialog if empty)"=w284, "format (%s)"="%s" ("format (%.3f)"), "1D data"=w280, "append to file? (new file:F)"=TRUE) -> ("new file path (Not A Path if cancelled)"=w282:path, "error out"=w281:errorcluster)  [unwired: 10 in]
          }
          frame True {
          }
        }
        n153 = Decimal String To Number(string=w264) -> (number=w249:i32)  [unwired: 2 in, 1 out]
        n154 = Decimal String To Number(string=w263) -> (number=w248:i32)  [unwired: 2 in, 1 out]
        n155 = Reshape Array(w252, 30 ("dimension size")) -> (w250:dbl[])
        n156 = Build Array (concatenate)(w249, w248, w247, w250) -> (w245:dbl[])
        n157 = call-poly <vilib>:"Write Delimited Spreadsheet.vi"("file path (dialog if empty)"=w267, "format (%.3f)"="%.3f", "1D data"=w245, "append to file? (new file:F)"=TRUE, "error in (no error)"=w261) -> ()  [unwired: 9 in, 2 out]
      }
      frame "open heat switch" {
        # "40000 steps gives slightly more than 3 turns"
        # "Set speed.\nCommand = 42"
        # "https://www.zaber.com/manuals/T-NM#6-quick-command-reference"
        # "serial connection to heat switch is opened automatically with VISA write"
        n158 = call <instrlib>:"Write Command.vi"("Request"=T2 {"Device Number"=1, "Command"=42, "Data"=300, "Response Count"=1}, "VISA resource name"=refnum<visa-resource-name> "COM4") -> ("VISA resource name out"=w293:refnum<visa-resource-name>)  [unwired: 7 in, 2 out]
        n159 = call <instrlib>:"Write Command.vi"("Request"=T2 {"Device Number"=1, "Command"=21, "Data"=40000, "Response Count"=1}, "VISA resource name"=w293) -> ()  [unwired: 7 in, 3 out]
        n160 = local write "Ramp Status"("Opening heat switch button pushed! Nothing is connected..." ("Ramp Status")) -> ()
      }
      frame "close heat switch" {
        # "40000 steps gives slightly more than 3 turns"
        # "Set speed.\nCommand = 42"
        # "https://www.zaber.com/manuals/T-NM#6-quick-command-reference"
        n161 = call <instrlib>:"Write Command.vi"("Request"=T2 {"Device Number"=1, "Command"=42, "Data"=300, "Response Count"=1}, "VISA resource name"=refnum<visa-resource-name> "COM4") -> ("VISA resource name out"=w298:refnum<visa-resource-name>)  [unwired: 7 in, 2 out]
        n162 = call <instrlib>:"Write Command.vi"("Request"=T2 {"Device Number"=1, "Command"=21, "Data"=-47000, "Response Count"=1}, "VISA resource name"=w298) -> ()  [unwired: 7 in, 3 out]
      }
      frame "initialize ramp up" {
        w304 = u16 1 items=["Manual Off", "Manual On", "Alarms"] ("Relay Mode (0:Off)")
        w305 = u16 1 items=["Relay 1"=1, "Relay 2"=2] ("Relay (1:Relay 1)")
        w309 = u16 3 items=["31.6 uA", "100 uA", "316 uA", "1.00 mA", "3.16 mA", "10.0 mA", "31.6 mA", "100 mA"] ("Maximum Heater Range (0: 31.6 uA)")
        w320 = u16 2 items=["Closed Loop PID", "Zone Tuning", "Open Loop", "Off"] ("Control Mode (0: Closed Loop PID)")
        # "turn relay on to change to low\nresistance in series with magnet"
        n163 = local read "Ramp up step size (mA)"() -> (w315:dbl)
        n164 = local read "magnet ramp resistance ohms"() -> (w307:dbl)
        n165 = disable-structure shown="Disabled" {
          frame Disabled {
            w327 = u16 1 items=["Off", "On", "Alarms", "Sample Heater Zone", "Warmup Heater Zone"] ("Relay Mode (0: Off)")
            w337 = u16 0 items=["sample heater", "output 1 (warm-up heater) ", "output 2 (analog/still)"] ("Output (0: sample heater)")
            w333 = u16 0 items=["unipolar", "bipolar"] ("polarity")
            w331 = u16 2 items=["off", "monitor out", "open loop (manual)", "zone", "still", "closed loop (PID)", "warmup"] ("mode")
            w330 = u16 0 items=["sample heater", "output 1 (warm-up heater) ", "output 2 (analog/still)"] ("Output (0: sample heater)")
            # "Start the magnet ramping up. Check whether starting ramp from 0 (what if labview crashes while\nmagnet is ramping up?)"
            n166 = local read "Ramp up step size (mA)"() -> (w342:dbl)
            n167 = local read "ls370"() -> (w324:refnum<visa-resource-name>)
            n168 = call <instrlib>:"Heater Output.vi"("VISA resource name"=w324) -> ("VISA resource name out"=w323:refnum<visa-resource-name>, "Heater Output"=w321:dbl, "error out"=w322:errorcluster)  [unwired: 12 in]
            n169 = Divide(x=w342, y=100.0) -> (x/y=w341:dbl)
            n170 = Less Or Equal?(x=w321, y=w341) -> (x <= y?=w343:bool)
            n171 = Select(t=0.0, s=w343, f=w321) -> (s? t:f=w329:dbl)
            n172 = local read "Heater Range Set"() -> (w328:u16)
            n173 = call <instrlib>:"configure heater output.vi"("VISA resource name"=w323, "power up enable"=FALSE, "polarity"=w333, "delay"=0, "Output (0: sample heater)"=w330, "mode"=w331, "error in (no error)"=w322, "input/channel"="A", "filter"=FALSE) -> ("VISA resource name out"=w338:refnum<visa-resource-name>, "error out"=w339:errorcluster)  [unwired: 5 in]
            n174 = call <instrlib>:"Configure Control Parameters.vi"("VISA resource name"=w338, "Output (0: sample heater)"=w337, "Manual Output (0.000%)"=w329, "Heater Range (0: Off)"=w328, "error in (no error)"=w339) -> ("VISA resource name out"=w326:refnum<visa-resource-name>, "error out"=w325:errorcluster)  [unwired: 9 in]
            n175 = call <instrlib>:"Configure Relays.vi"("Relay Mode (0: Off)"=w327, "error in (no error)"=w325, "VISA resource name"=w326) -> ()  [unwired: 7 in, 2 out]
          }
          frame Enabled {
          }
        }
        n176 = local read "ls370"() -> (w318:refnum<visa-resource-name>)
        n177 = call <instrlib>:"Heater Output.vi"("VISA resource name"=w318) -> ("VISA resource name out"=w310:refnum<visa-resource-name>, "Heater Output"=w319:dbl)  [unwired: 12 in, 1 out]
        n178 = Divide(x=w315, y=100.0) -> (x/y=w316:dbl)
        n179 = local write "Magnet resistance ohms"(w307) -> ()
        n180 = Less Or Equal?(x=w319, y=w316) -> (x <= y?=w314:bool)
        n181 = Select(t=0.0, s=w314, f=w319) -> (s? t:f=w308:dbl)
        n182 = local read "Heater Range Set"() -> (w312:u16)
        n183 = call <instrlib>:"Config Control Mode.vi"("VISA resource name"=w310, "Control Mode (0: Closed Loop PID)"=w320, "Maximum Heater Range (0: 31.6 uA)"=w309) -> ("VISA resource name out"=w311:refnum<visa-resource-name>)  [unwired: 11 in, 1 out]
        n184 = local read "Gain(P)"() -> (w303:dbl)
        n185 = local read "Reset(I)"() -> (w302:dbl)
        n186 = local read "Rate(D)"() -> (w301:dbl)
        n187 = call <instrlib>:"Config Control Parameters.vi"("VISA resource name"=w311, "Manual Output (0.000%)"=w308, "Heater Range (0: Off)"=w312, "Gain(P) (10.000)"=w303, "Reset(I) (20)"=w302, "Rate(D) (0)"=w301) -> ()  [unwired: 8 in, 2 out]
        n188 = local read "ls350"() -> (w306:refnum<visa-resource-name>)
        n189 = call <instrlib>:"Configure Relay.vi"("VISA resource name"=w306, "Relay (1:Relay 1)"=w305, "Relay Mode (0:Off)"=w304) -> ()  [unwired: 11 in, 2 out]
      }
      frame "set up autoramp times" {
        n190 = local read "current time"() -> (w346:timestamp)
        n191 = local read "ramp start time"() -> (w345:timestamp)
        n192 = Greater?(x=w346, y=w345) -> (0:w347:bool)
        n193 = case shown="True" w347 {
          frame True {
            n194 = Get Date/Time In Seconds() -> (seconds since 1Jan1904=w381:timestamp)
            n195 = local read "Ramp down rate (mA/s)"() -> (w360:dbl)
            n196 = local read "Max current (A)"() -> (w367:dbl)
            n197 = local read "Ramp up rate (mA/s)"() -> (w364:dbl)
            n198 = local read "Timeout (ms)"() -> (w379:i32)
            n199 = local read "Timeout (ms)"() -> (w374:i32)
            n200 = local read "Max current (A)"() -> (w361:dbl)
            n201 = Add(x=w381, y=10.0) -> (x+y=w354:timestamp)
            n202 = local write "ramp start time"(w354) -> ()
            n203 = Divide(x=w379, y=1000) -> (x/y=w377:dbl)
            n204 = Divide(x=w374, y=1000) -> (x/y=w376:dbl)
            n205 = Multiply(x=w367, y=1000.0) -> (x*y=w365:dbl)
            n206 = Multiply(x=w361, y=1000.0) -> (x*y=w363:dbl)
            n207 = Divide(x=w365, y=w364) -> (x/y=w352:dbl)
            n208 = Multiply(x=w364, y=w377) -> (x*y=w369:dbl)
            n209 = Multiply(x=w360, y=w376) -> (x*y=w368:dbl)
            n210 = Divide(x=w363, y=w360) -> (x/y=w349:dbl)
            n211 = Divide(x=w368, y=10.0) -> (x/y=w371:dbl)
            n212 = Divide(x=w369, y=10.0) -> (x/y=w370:dbl)
            n213 = local write "Ramp up step size (mA)"(w369) -> ()
            n214 = local write "Ramp down step size (mA)"(w368) -> ()
            n215 = local write "Ramp down step size (%)"(w371) -> ()
            n216 = Divide(x=w352, y=60.0) -> (x/y=w353:dbl)
            n217 = local write "Ramp up step size (%)"(w370) -> ()
            n218 = Divide(x=w349, y=60.0) -> (x/y=w350:dbl)
            n219 = local write "ramp up time (min)"(w353) -> ()
            n220 = local write "ramp down time (min)"(w350) -> ()
            n221 = local read "soak time (minutes)"() -> (w359:dbl)
            n222 = local write "Ramp Status"("Current time is greater than Start Time! Starting ramp in 10 seconds" ("AutoRamp Status")) -> ()
            n223 = Multiply(x=w359, y=60.0) -> (x*y=w357:dbl)
            n224 = Add(x=w357, y=w352) -> (x+y=w355:dbl)
            n225 = Add(x=w355, y=w354) -> (x+y=w356:timestamp)
            n226 = local write "ramp down start time"(w356) -> ()
          }
          frame False {
            n227 = local read "Ramp down rate (mA/s)"() -> (w400:dbl)
            n228 = local read "Max current (A)"() -> (w407:dbl)
            n229 = local read "Ramp up rate (mA/s)"() -> (w404:dbl)
            n230 = local read "Timeout (ms)"() -> (w419:i32)
            n231 = local read "Timeout (ms)"() -> (w414:i32)
            n232 = local read "Max current (A)"() -> (w401:dbl)
            n233 = Divide(x=w419, y=1000) -> (x/y=w417:dbl)
            n234 = Multiply(x=w407, y=1000.0) -> (x*y=w405:dbl)
            n235 = Divide(x=w414, y=1000) -> (x/y=w416:dbl)
            n236 = Multiply(x=w401, y=1000.0) -> (x*y=w403:dbl)
            n237 = Divide(x=w405, y=w404) -> (x/y=w390:dbl)
            n238 = Multiply(x=w404, y=w417) -> (x*y=w409:dbl)
            n239 = Multiply(x=w400, y=w416) -> (x*y=w408:dbl)
            n240 = Divide(x=w403, y=w400) -> (x/y=w387:dbl)
            n241 = Divide(x=w390, y=60.0) -> (x/y=w391:dbl)
            n242 = Divide(x=w408, y=10.0) -> (x/y=w411:dbl)
            n243 = Divide(x=w409, y=10.0) -> (x/y=w410:dbl)
            n244 = local write "Ramp down step size (mA)"(w408) -> ()
            n245 = local write "Ramp up step size (mA)"(w409) -> ()
            n246 = local write "ramp up time (min)"(w391) -> ()
            n247 = local write "Ramp down step size (%)"(w411) -> ()
            n248 = local write "Ramp up step size (%)"(w410) -> ()
            n249 = Divide(x=w387, y=60.0) -> (x/y=w388:dbl)
            n250 = local write "ramp down time (min)"(w388) -> ()
            n251 = local read "soak time (minutes)"() -> (w399:dbl)
            n252 = local read "delay after ramp down (min)"() -> (w384:dbl)
            n253 = local write "Ramp Status"("Waiting for ramp to start..." ("AutoRamp Status")) -> ()
            n254 = local read "ramp start time"() -> (w396:timestamp)
            n255 = Multiply(x=w399, y=60.0) -> (x*y=w397:dbl)
            n256 = Add(x=w397, y=w390) -> (x+y=w395:dbl)
            n257 = Add(x=w395, y=w396) -> (x+y=w394:timestamp)
            n258 = Multiply(x=w384, y=60.0) -> (x*y=w385:dbl)
            n259 = Add(x=w394, y=w387) -> (x+y=w393:timestamp)
            n260 = local write "ramp down start time"(w394) -> ()
            n261 = Add(x=w393, y=w385) -> (x+y=w392:timestamp)
            n262 = local write "ramp finish time"(w392) -> ()
          }
        }
      }
      frame "Calculate ramp time" {
        n263 = local read "Ramp down rate (mA/s)"() -> (w438:dbl)
        n264 = local read "Max current (A)"() -> (w445:dbl)
        n265 = local read "Ramp up rate (mA/s)"() -> (w442:dbl)
        n266 = local read "Timeout (ms)"() -> (w457:i32)
        n267 = local read "Timeout (ms)"() -> (w452:i32)
        n268 = local read "Max current (A)"() -> (w439:dbl)
        n269 = Divide(x=w457, y=1000) -> (x/y=w455:dbl)
        n270 = Multiply(x=w445, y=1000.0) -> (x*y=w443:dbl)
        n271 = Divide(x=w452, y=1000) -> (x/y=w454:dbl)
        n272 = Multiply(x=w439, y=1000.0) -> (x*y=w441:dbl)
        n273 = Divide(x=w443, y=w442) -> (x/y=w428:dbl)
        n274 = Multiply(x=w442, y=w455) -> (x*y=w447:dbl)
        n275 = Multiply(x=w438, y=w454) -> (x*y=w446:dbl)
        n276 = Divide(x=w441, y=w438) -> (x/y=w425:dbl)
        n277 = Divide(x=w446, y=10.0) -> (x/y=w449:dbl)
        n278 = Divide(x=w447, y=10.0) -> (x/y=w448:dbl)
        n279 = local write "Ramp down step size (mA)"(w446) -> ()
        n280 = local write "Ramp up step size (mA)"(w447) -> ()
        n281 = Divide(x=w425, y=60.0) -> (x/y=w426:dbl)
        n282 = local write "Ramp down step size (%)"(w449) -> ()
        n283 = local write "Ramp up step size (%)"(w448) -> ()
        n284 = local write "ramp down time (min)"(w426) -> ()
        n285 = Divide(x=w428, y=60.0) -> (x/y=w429:dbl)
        n286 = local write "ramp up time (min)"(w429) -> ()
        n287 = local read "soak time (minutes)"() -> (w437:dbl)
        n288 = local read "delay after ramp down (min)"() -> (w423:dbl)
        n289 = Multiply(x=w437, y=60.0) -> (x*y=w435:dbl)
        n290 = Add(x=w435, y=w428) -> (x+y=w433:dbl)
        n291 = Add(x=w433, y=w425) -> (x+y=w434:dbl)
        n292 = Multiply(x=60.0, y=w423) -> (x*y=w422:dbl)
        n293 = Add(x=w434, y=w422) -> (x+y=w432:dbl)
        n294 = Divide(x=w432, y=60.0) -> (x/y=w430:dbl)
        n295 = local write "cycle time (min)"(w430) -> ()
      }
      frame "autoramp" {
        n296 = local read "current time"() -> (w460:timestamp)
        n297 = local read "ramp start time"() -> (w459:timestamp)
        n298 = Greater?(x=w460, y=w459) -> (0:w458:bool)
        n299 = case shown="True" w458 {
          frame False {
            n300 = local write "Ramp Status"("waiting for ramp start time" ("AutoRamp Status")) -> ()
          }
          frame True {
            n301 = local read "ramp down start time"() -> (w464:timestamp)
            n302 = local read "current time"() -> (w463:timestamp)
            n303 = Greater?(x=w463, y=w464) -> (0:w462:bool)
            n304 = case shown="False" w462 {
              frame False {
                n305 = local read "Max current (A)"() -> (w466:dbl)
                n306 = local read "Magnet Current (A)"() -> (w467:dbl)
                n307 = Greater Or Equal?(x=w467, y=w466) -> (x >= y?=w465:bool)
                n308 = case shown="False" w465 {
                  frame False {
                    n309 = local read "Ramp Magnet Up"() -> (w470:bool)
                    n310 = Equal?(x=w470, y=TRUE) -> (x = y?=w468:bool)
                    n311 = case shown="False" w468 {
                      frame False {
                        n312 = property on="Ramp Magnet Up" class="Bool (strict)"("Val(Sgnl)"=TRUE ("Value (Signaling)")) -> ()  [unwired: 2 in, 2 out]
                        n313 = property on="Heat Switch" class="Bool (strict)"("Val(Sgnl)"=TRUE ("Value (Signaling)")) -> ()  [unwired: 2 in, 2 out]
                      }
                      frame True {
                      }
                    }
                    n314 = local write "Ramp Status"("ramping up" ("AutoRamp Status")) -> ()
                  }
                  frame True {
                    n315 = local write "Ramp Magnet Up"(FALSE ("Auto-Ramp")) -> ()
                    n316 = local write "Ramp Status"("soaking" ("AutoRamp Status")) -> ()
                  }
                }
              }
              frame True {
                n317 = local read "Max current (A)"() -> (w477:dbl)
                n318 = local read "Magnet Current (A)"() -> (w478:dbl)
                n319 = Greater Or Equal?(x=w478, y=w477) -> (x >= y?=w476:bool)
                n320 = case shown="True" w476 {
                  frame False {
                    n321 = local read "Magnet Current (A)"() -> (w481:dbl)
                    n322 = local read "Ramp down step size (mA)"() -> (w483:dbl)
                    n323 = local write "Ramp Status"("ramping down" ("AutoRamp Status")) -> ()
                    n324 = Multiply(x=w481, y=1000.0) -> (x*y=w479:dbl)
                    n325 = Greater Or Equal?(x=w479, y=w483) -> (x >= y?=w482:bool)
                    n326 = case shown="False" w482 {
                      frame False {
                        n327 = local write "Auto-Ramp"(FALSE ("Auto-Ramp")) -> ()
                      }
                      frame True {
                      }
                    }
                  }
                  frame True {
                    n328 = property on="Ramp Magnet Down" class="Bool (strict)"("Val(Sgnl)"=TRUE ("Value (Signaling)")) -> ()  [unwired: 2 in, 2 out]
                    n329 = property on="Heat Switch" class="Bool (strict)"("Val(Sgnl)"=FALSE ("Value (Signaling)")) -> ()  [unwired: 2 in, 2 out]
                    n330 = local write "Ramp Status"("ramping down" ("Ramp Status")) -> ()
                  }
                }
              }
            }
          }
        }
      }
      frame "check ramp state" {
        n331 = local read "Ramp State"() -> (w490:u16)
        n332 = case shown="2" w490 {
          tunnel: w489 -> [_ _ w547 _ _ _ _]
          frame 0 {
            # "Ramp Up"
            # "Steps:\n1. Increment magnet until max value is reached\n2. Change Ramp State to Soak (hold)"
            n333 = local read "Magnet Current (A)"() -> (w493:dbl)
            n334 = local read "Max current (A)"() -> (w492:dbl)
            n335 = Greater Or Equal?(x=w493, y=w492) -> (x >= y?=w491:bool)
            n336 = case shown="False" w491 {
              frame False {
                # "step size amps"
                # "lakeshore out %"
                # "lakeshore out current"
                # "kepco in voltage"
                # "kepco out voltage"
                # "increment magnet"
                n337 = local read "Heater Range Actual"() -> (w507:u16)
                n338 = local read "Ramp up rate (mA/s)"() -> (w515:dbl)
                n339 = local read "Timeout (ms)"() -> (w514:i32)
                n340 = Divide(x=w514, y=1000) -> (x/y=w512:dbl)
                n341 = local read "Magnet resistance ohms"() -> (w504:dbl)
                n342 = Multiply(x=w515, y=w512) -> (x*y=w505:dbl)
                n343 = local write "Ramp up step size (mA)"(w505) -> ()
                n344 = Divide(x=w505, y=1000.0) -> (x/y=w498:dbl)
                n345 = local read "lakeshore output %"() -> (w511:dbl)
                n346 = Multiply(x=w498, y=w504) -> (x*y=w503:dbl)
                n347 = local read "Heater Range Set"() -> (w508:u16)
                n348 = local read "Gain(P)"() -> (w496:dbl)
                n349 = local read "Reset(I)"() -> (w495:dbl)
                n350 = local read "Rate(D)"() -> (w494:dbl)
                n351 = Divide(x=w503, y=2.0) -> (x/y=w501:dbl)
                n352 = local read "ls370"() -> (w510:refnum<visa-resource-name>)
                n353 = Divide(x=w501, y=10.0) -> (x/y=w499:dbl)
                n354 = case shown="1" w507 {
                  tunnel: [w516 w519 w522 w525 w528 w531 w534 w537 w541] -> w506
                  tunnel: w499 -> [w517 w520 w523 w526 w529 w532 w535 w538 w540]
                  frame 2 {
                    n355 = Divide(x=w517, y=0.001) -> (x/y=w516:dbl)
                  }
                  frame 3 {
                    n356 = Divide(x=w520, y=0.00316) -> (x/y=w519:dbl)
                  }
                  frame 4 {
                    n357 = Divide(x=w523, y=0.01) -> (x/y=w522:dbl)
                  }
                  frame 5 {
                    n358 = Divide(x=w526, y=0.0316) -> (x/y=w525:dbl)
                  }
                  frame 6 {
                    n359 = Divide(x=w529, y=0.1) -> (x/y=w528:dbl)
                  }
                  frame 7 {
                    n360 = Divide(x=w532, y=0.316) -> (x/y=w531:dbl)
                  }
                  frame 8 {
                    n361 = Divide(x=w535, y=1.0) -> (x/y=w534:dbl)
                  }
                  frame 0, Default {
                    n362 = Multiply(x=w538, y=0.0) -> (x*y=w537:dbl)
                  }
                  frame 1 {
                    n363 = Divide(x=w540, y=0.000316) -> (x/y=w541:dbl)
                  }
                }
                n364 = Add(x=w511, y=w506) -> (x+y=w509:dbl)
                n365 = call <instrlib>:"Config Control Parameters.vi"("VISA resource name"=w510, "Manual Output (0.000%)"=w509, "Heater Range (0: Off)"=w508, "Gain(P) (10.000)"=w496, "Reset(I) (20)"=w495, "Rate(D) (0)"=w494) -> ()  [unwired: 8 in, 2 out]
              }
              frame True {
                w544 = u16 1 items=["Ramp Up", "Soak (hold)", "Ramp Down", "Ramp up to Setpoint", "Closed Loop Feedback", "Ramp down from Setpoint", "Magnet off"] ("Ramp State")
                n366 = local write "Ramp State"(w544) -> ()
                n367 = local write "Ramp Magnet Up"(FALSE ("Ramp Magnet Up")) -> ()
              }
            }
          }
          frame 1, Default {
            # "Soak (hold)"
            # "Steps:\n1. Do nothing! but indicate that magnet is on"
            n368 = local read "magnet ramp resistance ohms"() -> (w545:dbl)
            n369 = local write "Magnet resistance ohms"(w545) -> ()
          }
          frame 2 {
            # "Steps:\n1. Decrement magnet until min value is reached\n2. Change Ramp State to Magnet off"
            # "Ramp Down"
            n370 = local read "Ramp down step size (mA)"() -> (w549:dbl)
            n371 = local read "Magnet Current (A)"() -> (w551:dbl)
            n372 = Divide(x=w549, y=1000.0) -> (x/y=w550:dbl)
            n373 = Less Or Equal?(x=w551, y=w550) -> (x <= y?=w546:bool)
            n374 = case shown="True" w546 {
              tunnel: w547 -> [_ w610]
              frame False {
                # "step size amps"
                # "lakeshore out %"
                # "lakeshore out current"
                # "kepco in voltage"
                # "kepco out voltage"
                # "decrement magnet"
                n375 = local read "Heater Range Actual"() -> (w563:u16)
                n376 = local read "Ramp down rate (mA/s)"() -> (w555:dbl)
                n377 = local read "Timeout (ms)"() -> (w556:i32)
                n378 = Divide(x=w556, y=1000) -> (x/y=w558:dbl)
                n379 = local read "Magnet resistance ohms"() -> (w566:dbl)
                n380 = Multiply(x=w555, y=w558) -> (x*y=w565:dbl)
                n381 = local write "Ramp down step size (mA)"(w565) -> ()
                n382 = Divide(x=w565, y=1000.0) -> (x/y=w572:dbl)
                n383 = local read "lakeshore output %"() -> (w559:dbl)
                n384 = Multiply(x=w572, y=w566) -> (x*y=w567:dbl)
                n385 = local read "Heater Range Set"() -> (w562:u16)
                n386 = Divide(x=w567, y=2.0) -> (x/y=w569:dbl)
                n387 = local read "ls370"() -> (w560:refnum<visa-resource-name>)
                n388 = local read "Gain(P)"() -> (w554:dbl)
                n389 = local read "Reset(I)"() -> (w553:dbl)
                n390 = local read "Rate(D)"() -> (w552:dbl)
                n391 = Divide(x=w569, y=10.0) -> (x/y=w571:dbl)
                n392 = case shown="1" w563 {
                  tunnel: [w574 w577 w580 w583 w586 w589 w592 w595 w599] -> w564
                  tunnel: w571 -> [w575 w578 w581 w584 w587 w590 w593 w596 w598]
                  frame 2 {
                    n393 = Divide(x=w575, y=0.001) -> (x/y=w574:dbl)
                  }
                  frame 3 {
                    n394 = Divide(x=w578, y=0.00316) -> (x/y=w577:dbl)
                  }
                  frame 4 {
                    n395 = Divide(x=w581, y=0.01) -> (x/y=w580:dbl)
                  }
                  frame 5 {
                    n396 = Divide(x=w584, y=0.0316) -> (x/y=w583:dbl)
                  }
                  frame 6 {
                    n397 = Divide(x=w587, y=0.1) -> (x/y=w586:dbl)
                  }
                  frame 7 {
                    n398 = Divide(x=w590, y=0.316) -> (x/y=w589:dbl)
                  }
                  frame 8 {
                    n399 = Divide(x=w593, y=1.0) -> (x/y=w592:dbl)
                  }
                  frame 0, Default {
                    n400 = Multiply(x=w596, y=0.0) -> (x*y=w595:dbl)
                  }
                  frame 1 {
                    n401 = Divide(x=w598, y=0.000316) -> (x/y=w599:dbl)
                  }
                }
                n402 = Subtract(x=w559, y=w564) -> (x-y=w561:dbl)
                n403 = call <instrlib>:"Config Control Parameters.vi"("VISA resource name"=w560, "Manual Output (0.000%)"=w561, "Heater Range (0: Off)"=w562, "Gain(P) (10.000)"=w554, "Reset(I) (20)"=w553, "Rate(D) (0)"=w552) -> ()  [unwired: 8 in, 2 out]
              }
              frame True {
                n404 = local read "delay after ramp down (min)"() -> (w603:dbl)
                n405 = local read "Timeout (ms)"() -> (w608:i32)
                n406 = Divide(x=w608, y=1000) -> (x/y=w606:dbl)
                n407 = Multiply(x=w603, y=60.0) -> (x*y=w602:dbl)
                n408 = Divide(x=w602, y=w606) -> (x/y=w609:dbl)
                n409 = local read "counter"() -> (w604:dbl)
                n410 = Greater Or Equal?(x=w604, y=w609) -> (x >= y?=w605:bool)
                n411 = case shown="True" w605 {
                  tunnel: w610 -> [_ w624]
                  tunnel: w604 -> [w611 _]
                  frame False {
                    n412 = Increment(x=w611) -> (x+1=w612:dbl)
                    n413 = local write "counter"(w612) -> ()
                  }
                  frame True {
                    w620 = u16 0 items=["Manual Off", "Manual On", "Alarms"] ("Relay Mode (0:Off)")
                    w621 = u16 1 items=["Relay 1"=1, "Relay 2"=2] ("Relay (1:Relay 1)")
                    w623 = u16 0 items=["Off", "31.6 uA", "100 uA", "316 uA", "1.00 mA", "3.16 mA", "10.0 mA", "31.6 mA", "100 mA"] ("Heater Range Set")
                    # "Turn heater off, set\nmanual out to zero"
                    n414 = local write "Ramp Status"("Ramp finished. " ("AutoRamp Status")) -> ()
                    n415 = local read "End of Ramp Temp Control"() -> (w625:bool)
                    n416 = local read "Gain(P)"() -> (w616:dbl)
                    n417 = local read "Reset(I)"() -> (w615:dbl)
                    n418 = local read "Rate(D)"() -> (w614:dbl)
                    n419 = local write "Ramp Magnet Down"(FALSE ("Auto-Ramp")) -> ()
                    n420 = local read "ls370"() -> (w617:refnum<visa-resource-name>)
                    n421 = call <instrlib>:"Config Control Parameters.vi"("VISA resource name"=w617, "Gain(P) (10.000)"=w616, "Reset(I) (20)"=w615, "Rate(D) (0)"=w614) -> ()  [unwired: 10 in, 2 out]
                    n422 = local read "ls350"() -> (w622:refnum<visa-resource-name>)
                    n423 = local read "magnet control resistance ohms"() -> (w613:dbl)
                    n424 = call <instrlib>:"Configure Relay.vi"("VISA resource name"=w622, "Relay (1:Relay 1)"=w621, "Relay Mode (0:Off)"=w620) -> ()  [unwired: 11 in, 2 out]
                    n425 = case shown="True" w625 {
                      tunnel: w624 -> [_ w631]
                      frame False {
                        w629 = u16 6 items=["Ramp Up", "Soak (hold)", "Ramp Down", "Ramp up to Setpoint", "Closed Loop Feedback", "Ramp down from Setpoint", "Magnet off"] ("Ramp State")
                        n426 = local write "Manual temp control"(FALSE ("temp control?")) -> ()
                        n427 = local write "Ramp State"(w629) -> ()
                      }
                      frame True {
                        n428 = local write "Ramp Status"("Turning on PID FEEDBACK\n" ("Arduino Response 2")) -> ()
                        n429 = Enqueue Element(queue=w631, element="turn on PID feedback") -> ()  [unwired: 2 in, 3 out]
                      }
                    }
                    n430 = local write "Heater Range Set"(w623) -> ()
                    n431 = local write "Magnet resistance ohms"(w613) -> ()
                    n432 = local read "Arduino"() -> (w619:refnum<visa-resource-name>)
                    n433 = VISA Write(VISA resource name=w619, write buffer="r") -> ()  [unwired: 1 in, 3 out]
                  }
                }
              }
            }
          }
          frame 3 {
            # "Ramp up to Setpoint"
          }
          frame 4 {
            # "Steps:\n1. Keep an eye on magnet value. If magnet runs out, turn it off"
            # "Closed Loop Feedback"
            n434 = local read "Magnet Current (A)"() -> (w635:dbl)
            n435 = Less Or Equal?(x=w635, y=0.003) -> (x <= y?=w633:bool)
            n436 = case shown="False" w633 {
              frame False {
                n437 = local write "counter 2"(0.0 ("counter 2")) -> ()
                n438 = local write "Ramp Status"("controlling..." ("Ramp Status")) -> ()
              }
              frame True {
                n439 = local read "counter 2"() -> (w639:dbl)
                n440 = Greater Or Equal?(x=w639, y=300.0) -> (x >= y?=w638:bool)
                n441 = case shown="False" w638 {
                  tunnel: w639 -> [w641 _]
                  frame False {
                    n442 = Increment(x=w641) -> (x+1=w642:dbl)
                    n443 = local write "counter 2"(w642) -> ()
                  }
                  frame True {
                    w643 = u16 6 items=["Ramp Up", "Soak (hold)", "Ramp Down", "Ramp up to Setpoint", "Closed Loop Feedback", "Ramp down from Setpoint", "Magnet off"] ("Ramp State")
                    w660 = u16 0 items=["Off", "31.6 uA", "100 uA", "316 uA", "1.00 mA", "3.16 mA", "10.0 mA", "31.6 mA", "100 mA"] ("Heater Range (0: Off)")
                    w649 = u16 0 items=["unipolar", "bipolar"] ("polarity")
                    w647 = u16 0 items=["off", "monitor out", "open loop (manual)", "zone", "still", "closed loop (PID)", "warmup"] ("mode")
                    w654 = u16 0 items=["sample heater", "output 1 (warm-up heater) ", "output 2 (analog/still)"] ("Output (0: sample heater)")
                    n444 = local read "ls370"() -> (w656:refnum<visa-resource-name>)
                    n445 = Get Date/Time String() -> (time string=w645:string)  [unwired: 3 in, 1 out]
                    n446 = local write "Ramp State"(w643) -> ()
                    n447 = call <instrlib>:"Configure Setpoint.vi"("Setpoint (0.00000E+0)"=0.01, "VISA resource name"=w656) -> ("VISA resource name out"=w657:refnum<visa-resource-name>)  [unwired: 8 in, 1 out]
                    n448 = Concatenate Strings("magnet ran out at " ("Ramp Status"), w645) -> (w646:string)
                    n449 = local read "control channel"() -> (w659:string)
                    n450 = local write "Ramp Status"(w646) -> ()
                    n451 = local write "Heater Range Set"(w660) -> ()
                    n452 = call <instrlib>:"configure heater output.vi"("VISA resource name"=w657, "power up enable"=FALSE, "polarity"=w649, "delay"=0, "Output (0: sample heater)"=w654, "mode"=w647, "input/channel"=w659, "filter"=FALSE) -> ("VISA resource name out"=w652:refnum<visa-resource-name>, "error out"=w653:errorcluster)  [unwired: 6 in]
                    n453 = call <instrlib>:"Configure Control Parameters.vi"("VISA resource name"=w652, "Output (0: sample heater)"=w654, "Manual Output (0.000%)"=0.0, "Heater Range (0: Off)"=w660, "error in (no error)"=w653) -> ()  [unwired: 9 in, 2 out]
                  }
                }
              }
            }
          }
          frame 5 {
            # "Ramp down from Setpoint"
            n454 = local read "Ramp down step size (mA)"() -> (w663:dbl)
            n455 = local read "Magnet Current (A)"() -> (w665:dbl)
            n456 = Divide(x=w663, y=1000.0) -> (x/y=w664:dbl)
            n457 = Less Or Equal?(x=w665, y=w664) -> (x <= y?=w661:bool)
            n458 = case shown="True" w661 {
              frame False {
                n459 = local read "ls370"() -> (w666:refnum<visa-resource-name>)
                n460 = call <instrlib>:"Get Setpoint.vi"("VISA resource name"=w666) -> ("Setpoint (0.00000E+0)"=w669:dbl)  [unwired: 8 in, 2 out]
                n461 = Greater Or Equal?(x=w669, y=0.01) -> (x >= y?=w667:bool)
                n462 = case shown="True" w667 {
                  frame False {
                  }
                  frame True {
                    w685 = u16 0 items=["sample heater", "output 1 (warm-up heater) ", "output 2 (analog/still)"] ("Output (0: sample heater)")
                    w677 = u16 0 items=["unipolar", "bipolar"] ("polarity")
                    w675 = u16 5 items=["off", "monitor out", "open loop (manual)", "zone", "still", "closed loop (PID)", "warmup"] ("mode")
                    w674 = u16 0 items=["sample heater", "output 1 (warm-up heater) ", "output 2 (analog/still)"] ("Output (0: sample heater)")
                    n463 = local read "control channel"() -> (w672:string)
                    n464 = local read "ls370"() -> (w682:refnum<visa-resource-name>)
                    n465 = local read "Heater Range Set"() -> (w673:u16)
                    n466 = call <instrlib>:"configure heater output.vi"("VISA resource name"=w682, "power up enable"=FALSE, "polarity"=w677, "delay"=0, "Output (0: sample heater)"=w674, "mode"=w675, "input/channel"=w672, "filter"=FALSE) -> ("VISA resource name out"=w680:refnum<visa-resource-name>, "error out"=w681:errorcluster)  [unwired: 6 in]
                    n467 = call <instrlib>:"Configure Control Parameters.vi"("VISA resource name"=w680, "Output (0: sample heater)"=w685, "Manual Output (0.000%)"=0.0, "Heater Range (0: Off)"=w673, "error in (no error)"=w681) -> ("VISA resource name out"=w683:refnum<visa-resource-name>, "error out"=w684:errorcluster)  [unwired: 9 in]
                    n468 = call <instrlib>:"Configure Setpoint.vi"("error in (no error)"=w684, "Setpoint (0.00000E+0)"=0.001, "Output (0: Sample Heater)"=w685, "VISA resource name"=w683) -> ()  [unwired: 6 in, 2 out]
                  }
                }
              }
              frame True {
                w690 = u16 0 items=["unipolar", "bipolar"] ("polarity")
                w691 = u16 0 items=["Off", "31.6 uA", "100 uA", "316 uA", "1.00 mA", "3.16 mA", "10.0 mA", "31.6 mA", "100 mA"] ("Heater Range Set")
                w692 = u16 6 items=["Ramp Up", "Soak (hold)", "Ramp Down", "Ramp up to Setpoint", "Closed Loop Feedback", "Ramp down from Setpoint", "Magnet off"] ("Ramp State")
                w696 = u16 0 items=["sample heater", "output 1 (warm-up heater) ", "output 2 (analog/still)"] ("Output (0: sample heater)")
                w694 = u16 0 items=["off", "monitor out", "open loop (manual)", "zone", "still", "closed loop (PID)", "warmup"] ("mode")
                n469 = local write "Ramp Status"("Ramp finished. " ("AutoRamp Status")) -> ()
                n470 = local read "control channel"() -> (w686:string)
                n471 = local read "ls370"() -> (w695:refnum<visa-resource-name>)
                n472 = call <instrlib>:"configure heater output.vi"("VISA resource name"=w695, "power up enable"=FALSE, "polarity"=w690, "delay"=0, "Output (0: sample heater)"=w696, "mode"=w694, "input/channel"=w686, "filter"=FALSE) -> ()  [unwired: 6 in, 2 out]
                n473 = local write "Ramp Magnet Down"(FALSE ("Auto-Ramp")) -> ()
                n474 = local write "Heater Range Set"(w691) -> ()
                n475 = local write "Ramp State"(w692) -> ()
              }
            }
          }
          frame 6 {
            # "Magnet off"
            n476 = local read "Heater Range Actual"() -> (w700:u16)
            n477 = Equal?(x=w700, y=u16 0) -> (x = y?=w698:bool)
            n478 = case shown="False" w698 {
              frame False {
                w701 = u16 0 items=["Off", "31.6 uA", "100 uA", "316 uA", "1.00 mA", "3.16 mA", "10.0 mA", "31.6 mA", "100 mA"] ("Heater Range Set")
                n479 = local write "Heater Range Set"(w701) -> ()
              }
              frame True {
              }
            }
          }
        }
      }
      frame "turn on PID feedback" {
        w707 = u16 4 items=["Ramp Up", "Soak (hold)", "Ramp Down", "Ramp up to Setpoint", "Closed Loop Feedback", "Ramp down from Setpoint", "Magnet off"] ("Ramp State")
        w711 = u16 3 items=["Off", "31.6 uA", "100 uA", "316 uA", "1.00 mA", "3.16 mA", "10.0 mA", "31.6 mA", "100 mA"] ("Heater Range (0: Off)")
        w714 = u16 3 items=["31.6 uA", "100 uA", "316 uA", "1.00 mA", "3.16 mA", "10.0 mA", "31.6 mA", "100 mA"] ("Maximum Heater Range (0: 31.6 uA)")
        w716 = u16 0 items=["Closed Loop PID", "Zone Tuning", "Open Loop", "Off"] ("Control Mode (0: Closed Loop PID)")
        # "1.1, 60, 15 for PID"
        n480 = local read "ls370"() -> (w717:refnum<visa-resource-name>)
        n481 = local read "magnet control resistance ohms"() -> (w702:dbl)
        n482 = local write "Magnet resistance ohms"(w702) -> ()
        n483 = local read "Gain(P)"() -> (w705:dbl)
        n484 = local read "Reset(I)"() -> (w704:dbl)
        n485 = local read "Rate(D)"() -> (w703:dbl)
        n486 = call <instrlib>:"Config Control Mode.vi"("VISA resource name"=w717, "Control Mode (0: Closed Loop PID)"=w716, "Heater Resistance (100.00)"=10000.0, "Maximum Heater Range (0: 31.6 uA)"=w714) -> ("VISA resource name out"=w713:refnum<visa-resource-name>, "error out"=w712:errorcluster)  [unwired: 10 in]
        n487 = local write "Heater Range Set"(w711) -> ()
        n488 = local write "Ramp State"(w707) -> ()
        n489 = local read "setpoint (K)"() -> (w708:dbl)
        n490 = call <instrlib>:"Config Control Parameters.vi"("VISA resource name"=w713, "Heater Range (0: Off)"=w711, "Gain(P) (10.000)"=w705, "Reset(I) (20)"=w704, "error in (no error)"=w712, "Rate(D) (0)"=w703) -> ("VISA resource name out"=w710:refnum<visa-resource-name>, "error out"=w709:errorcluster)  [unwired: 8 in]
        n491 = call <instrlib>:"Config Setpoint.vi"("VISA resource name"=w710, "Setpoint (0.00000E+0)"=w708, "error in (no error)"=w709) -> ()  [unwired: 11 in, 2 out]
        n492 = local write "counter 2"(0.0 ("counter 2")) -> ()
      }
      frame "Write LS372 Settings" {
        w718 = u16 1 items=["Kelvin"=1, "Ohms"=2] ("Preferred Units (2: Ohms)")
        n493 = local read "ls370"() -> (w726:refnum<visa-resource-name>)
        n494 = call <instrlib>:"Configure Input Sensor Range.vi"("VISA resource name"=w726, "Channel (1)"="Channel (1)", "Excitation Mode (0: Voltage)"="Excitation Mode (0: Voltage)", "Excitation Range (5: 200 uV / 100 pA)"="Excitation Range (5: 200 uV / 100 pA)", "Autorange (0: Autorange off)"="Autorange (0: Autorange off)", "Resistance Range (17: 200 kOhm)"="Resistance Range (17: 200 kOhm)", "Excitation  (T: On)"="Excitation  (T: On)", "Preferred Units (2: Ohms)"=w718, "Temperature Limit (0 Kelvin)"=0.0) -> ()  [unwired: 9 in, 2 out]
      }
      frame "Switch Warmup Heater" {
        # "0 for off\n1 for on"
        n495 = local write "Ramp Status"("warmup heater button pushed!" ("Ramp Status")) -> ()
        n496 = local read "ls350"() -> (w739:refnum<visa-resource-name>)
        n497 = call <instrlib>:"Configure Heater Output.vi"("VISA resource name"=w739, "Mode (0:Off)"="Mode (0:Off)", "Heater Output (1:1)"="Heater Output (1:1)", "Input (0:None)"="Input (0:None)", "Max Current (0:User Specified)"="Max Current (0:User Specified)", "Heater Out Display (1:Current)"="Heater Out Display (1:Current)", "Max User Current (2.000)"="Max User Current (2.000)", "Heater Resistance (1:25 Ohms)"="Heater Resistance (1:25 Ohms)") -> ("VISA resource name out"=w731:refnum<visa-resource-name>, "error out"=w730:errorcluster)  [unwired: 6 in]
        n498 = call <instrlib>:"Configure Output Range and Manual Value.vi"("VISA resource name"=w731, "Output (1:1)"="heater output", "Range (0:Off)"="warmup heater Range", "Manual Output (0.00 %)"="warmup heater output %", "error in (no error)"=w730) -> ()  [unwired: 9 in, 2 out]
      }
      frame "update PID values" {
        n499 = local read "Heater Range Actual"() -> (w742:u16)
        n500 = local read "lakeshore output %"() -> (w741:dbl)
        n501 = local read "ls370"() -> (w743:refnum<visa-resource-name>)
        n502 = local read "Gain(P)"() -> (w746:dbl)
        n503 = local read "Reset(I)"() -> (w745:dbl)
        n504 = local read "Rate(D)"() -> (w744:dbl)
        n505 = call <instrlib>:"Config Control Parameters.vi"("VISA resource name"=w743, "Manual Output (0.000%)"=w741, "Heater Range (0: Off)"=w742, "Gain(P) (10.000)"=w746, "Reset(I) (20)"=w745, "Rate(D) (0)"=w744) -> ()  [unwired: 8 in, 2 out]
        n506 = disable-structure shown="Disabled" {
          frame Disabled {
            n507 = local read "Gain(P)"() -> (w751:dbl)
            n508 = local read "Reset(I)"() -> (w750:dbl)
            n509 = local read "Rate(D)"() -> (w749:dbl)
            n510 = local read "ls370"() -> (w748:refnum<visa-resource-name>)
            n511 = Format Value(format string="%.;PID %.;%.3f,", value (0)=w751) -> (output string=w755:string)  [unwired: 1 in]
            n512 = Format Value(string ("")=w755, format string="%d,", value (0)=w750) -> (output string=w756:string)
            n513 = Format Value(string ("")=w756, format string="%d", value (0)=w749) -> (output string=w747:string)
            n514 = call "Serial Write_370.vi"("Write Buffer (\"\")"=w747, "VISA resource name"=w748) -> ()  [unwired: 7 in, 3 out]
          }
          frame Enabled {
          }
        }
      }
      frame "query HEMT voltages" {
        n515 = local read "Arduino"() -> (w765:refnum<visa-resource-name>)
        n516 = VISA Clear(VISA resource name=w765) -> (VISA resource name out=w764:refnum<visa-resource-name>)  [unwired: 1 in, 1 out]
        n517 = VISA Write(VISA resource name=w764, write buffer="v") -> (VISA resource name out=w767:refnum<visa-resource-name>)  [unwired: 1 in, 2 out]
        n518 = VISA Read(VISA resource name=w767, byte count=u32 1024) -> (read buffer=w763:string)  [unwired: 1 in, 3 out]
        n519 = Spreadsheet String To Array(delimiter (Tab)=",", format string="%f", spreadsheet string=w763) -> (array=w760:dbl[][])  [unwired: 1 in]
        n520 = Reshape Array(w760, 10 ("dimension size"), 3 ("dimension size")) -> (w757:dbl[][])
        n521 = local write "HEMT biases"(w757) -> ()
      }
      frame "query select HEMT voltages" {
        n522 = local read "Arduino"() -> (w777:refnum<visa-resource-name>)
        n523 = VISA Clear(VISA resource name=w777) -> (VISA resource name out=w776:refnum<visa-resource-name>)  [unwired: 1 in, 1 out]
        n524 = VISA Write(VISA resource name=w776, write buffer="A") -> (VISA resource name out=w779:refnum<visa-resource-name>)  [unwired: 1 in, 2 out]
        n525 = VISA Read(VISA resource name=w779, byte count=u32 1024) -> (read buffer=w775:string)  [unwired: 1 in, 3 out]
        n526 = Spreadsheet String To Array(delimiter (Tab)=",", format string="%f", spreadsheet string=w775) -> (array=w772:dbl[][])  [unwired: 1 in]
        n527 = Reshape Array(w772, 10 ("dimension size"), 3 ("dimension size")) -> (w769:dbl[][])
        n528 = local write "HEMT biases"(w769) -> ()
      }
      frame "query 1 hemt voltage" {
        # "hemt v counter \nstarts at 65 (A in ascii) \nand goes to 95, because we have\n30 voltages to read out."
        # "SEND THE arduino ascii characters starting with A (65). Each different character corresponds to a unique hemt voltage."
        n529 = local read "hemt v counter"() -> (w798:i32)
        n530 = local read "Arduino"() -> (w807:refnum<visa-resource-name>)
        n531 = Greater Or Equal?(x=w798, y=95) -> (x >= y?=w805:bool)
        n532 = VISA Clear(VISA resource name=w807) -> (VISA resource name out=w806:refnum<visa-resource-name>, error out=w801:errorcluster)  [unwired: 1 in]
        n533 = case shown="True" w805 {
          tunnel: w798 -> [w810 _]
          frame False {
            n534 = Increment(x=w810) -> (x+1=w811:i32)
            n535 = local write "hemt v counter"(w811) -> ()
          }
          frame True {
            n536 = local write "hemt v counter"(65 ("hemt v counter")) -> ()
          }
        }
        n537 = Type Cast(type="", x=w798) -> (*(type *) &x=w803:string)
        n538 = VISA Write(VISA resource name=w806, write buffer=w803, error in (no error)=w801) -> (VISA resource name out=w809:refnum<visa-resource-name>, error out=w800:errorcluster)  [unwired: 1 out]
        n539 = VISA Read(VISA resource name=w809, byte count=u32 1024, error in (no error)=w800) -> (read buffer=w793:string, error out=w781:errorcluster)  [unwired: 2 out]
        n540 = local write "error out"(w781) -> ()
        n541 = Subtract(x=w798, y=65) -> (x-y=w782:i32)
        n542 = local read "HEMT biases"() -> (w799:dbl[][])
        n543 = Decimal String To Number(string=w793) -> (number=w792:i32)  [unwired: 2 in, 1 out]
        n544 = Quotient & Remainder(x=w782, y=3) -> (x-y*floor(x/y)=w794:i32, floor(x/y)=w795:i32)
        n545 = Spreadsheet String To Array(delimiter (Tab)=",", format string="%s", spreadsheet string="A1vd, A1id, A1vg,A2vd, A2id, A2vg,A3vd, A3id, A3vg,A4vd, A4id, A4vg,A5vd, A5id, A5vg,B1vd, B1id, A1vg,B2vd, B2id, B2vg,B3vd, B3id, B3vg,B4vd, B4id, B4vg,B5vd, B5id, B5vg ", array type (2D Dbl)="") -> (array=w786:string[][])
        n546 = Replace Array Subset(array=w799, new element=w792, index (row)=w795, index (col)=w794) -> (w791:dbl[][])
        n547 = Index Array(array=w786, index (row)=0) -> (element=w784:string[])  [unwired: 1 in]
        n548 = local write "HEMT biases"(w791) -> ()
        n549 = Index Array(array=w784, index=w782) -> (element=→"element":string)
      }
      frame "close MUX relays" {
        n550 = local read "Arduino"() -> (w815:refnum<visa-resource-name>)
        n551 = VISA Write(VISA resource name=w815, write buffer="s") -> (error out=w813:errorcluster)  [unwired: 1 in, 2 out]
        n552 = local write "error out"(w813) -> ()
      }
      frame "open MUX relays" {
        n553 = local read "Arduino"() -> (w818:refnum<visa-resource-name>)
        n554 = VISA Write(VISA resource name=w818, write buffer="r") -> (error out=w816:errorcluster)  [unwired: 1 in, 2 out]
        n555 = local write "error out"(w816) -> ()
      }
      frame "read adc mag current" {
        n556 = local read "Arduino"() -> (w839:refnum<visa-resource-name>)
        n557 = VISA Clear(VISA resource name=w839) -> (VISA resource name out=w838:refnum<visa-resource-name>, error out=w821:errorcluster)  [unwired: 1 in]
        n558 = VISA Write(VISA resource name=w838, write buffer="c", error in (no error)=w821) -> (VISA resource name out=w841:refnum<visa-resource-name>, error out=w820:errorcluster)  [unwired: 1 out]
        n559 = VISA Read(VISA resource name=w841, byte count=u32 1024, error in (no error)=w820) -> (read buffer=w835:string, error out=w819:errorcluster)  [unwired: 2 out]
        n560 = local write "error out"(w819) -> ()
        n561 = Spreadsheet String To Array(delimiter (Tab)=",", format string="%f", spreadsheet string=w835) -> (array=w829:dbl[][])  [unwired: 1 in]
        "ADC0 outputs" <- w829
        n562 = Index Array(array=w829, index (row)=0, index (col)=0 ("disabled index (col)")) -> (element=w831:dbl)
        n563 = Index Array(array=w829, index (row)=0, index (col)=1 ("disabled index (col)")) -> (element=w824:dbl)
        "flow meter" <- w824
        n564 = Multiply(x=w831, y=0.00081473302) -> (x*y=→"adc magnet current (A)":dbl)
        n565 = Get Date/Time In Seconds() -> (seconds since 1Jan1904=w822:timestamp)
        n566 = Build Array(w824) -> (w826:dbl[])
        n567 = Bundle By Name("t0"=w822, "dt"=0.0, "Y"=w826) -> (→"Flow Meter":waveform(dbl))  [unwired: 1 in]
      }
    }
    n568 = Get Queue Status(queue=w50) -> (# elements in queue=w55:i32)  [unwired: 2 in, 7 out]
    n569 = Equal?(x=w55, y=0) -> (x = y?=w52:bool)
    n570 = local read "stopping"() -> (w53:bool)
    n571 = And(x=w53, y=w52) -> (x .and. y?=w51:bool)
  }
  n572 = while {
    tunnel: w47 -> [w846]
    tunnel: [w844] -> _
    stop <- w845 stop-if-true
    n573 = local read "Timeout (ms)"() -> (w843:i32)
    n574 = event shown="[1] \"Auto-Ramp\": Value Change" {
      selector: _ -> [_ _ _ _ _ _ _ _ _ _ _ _ _ _ _ _]
      dyn-events: _ -> [_ _ _ _ _ _ _ _ _ _ _ _ _ _ _ _]
      timeout: w843 -> [_ _ _ _ _ _ _ _ _ _ _ _ _ _ _ _]
      tunnel: w846 -> [w874 w898 _ w917 w923 w934 w944 w966 w968 w970 w973 w980 w982 w990 _ w1012]
      tunnel: [_ _ _ _ _ _ _ _ _ _ _ _ _ _ _ w1004] -> w844
      event Timeout {
        # "normal operating mode"
        n575 = event-data() -> ()  [unwired: 1 in, 3 out]
        n576 = local read "last record time"() -> (w854:dbl)
        n577 = Get Date/Time In Seconds() -> (seconds since 1Jan1904=w871:timestamp)
        n578 = To Double Precision Float(number=w871) -> (double precision float=w850:dbl)
        n579 = local read "read lakeshore sensors"() -> (w873:bool)
        n580 = Subtract(x=w850, y=w854) -> (x-y=w853:dbl)
        n581 = Greater Or Equal?(x=w853, y=10.0) -> (x >= y?=w851:bool)
        n582 = case shown="True" w873 {
          tunnel: w874 -> [w894 w896]
          tunnel: [w894 w895] -> w863
          frame False {
          }
          frame True {
            n583 = Enqueue Element(queue=w896, element="read temperature sensors") -> (queue out=w895:refnum<queue>)  [unwired: 2 in, 2 out]
          }
        }
        n584 = case shown="True" w851 {
          tunnel: [FALSE ("y") TRUE ("y")] -> w848
          tunnel: w850 -> [_ w876]
          frame False {
          }
          frame True {
            n585 = local write "last record time"(w876) -> ()
          }
        }
        n586 = And(x="Record Temps", y=w848) -> (x .and. y?=w870:bool)
        n587 = case shown="True" w870 {
          tunnel: w863 -> [w890 w893]
          tunnel: [w890 w892] -> w858
          tunnel: "record temps" ("element") -> [_ w891]
          frame False {
          }
          frame True {
            n588 = Enqueue Element(queue=w893, element=w891) -> (queue out=w892:refnum<queue>)  [unwired: 2 in, 2 out]
          }
        }
        n589 = And(x="auto-read HEMT voltages", y=w848) -> (x .and. y?=w856:bool)
        n590 = case shown="True" w856 {
          tunnel: w858 -> [w878 w883]
          tunnel: [w878 w880] -> w857
          tunnel: "query select HEMT voltages" ("element") -> [_ w882]
          tunnel: "record HEMT bias" ("element") -> [_ w879]
          frame False {
          }
          frame True {
            n591 = Enqueue Element(queue=w883, element=w882) -> (queue out=w881:refnum<queue>)  [unwired: 2 in, 2 out]
            n592 = Enqueue Element(queue=w881, element=w879) -> (queue out=w880:refnum<queue>)  [unwired: 2 in, 2 out]
          }
        }
        n593 = Get Date/Time In Seconds() -> (seconds since 1Jan1904=→"current time":timestamp)
        n594 = local read "Auto-Ramp"() -> (w864:bool)
        n595 = local read "Read ADC current"() -> (w859:bool)
        n596 = case shown="True" w859 {
          tunnel: [w884 w886] -> w861
          tunnel: "read adc mag current" -> [_ w887]
          tunnel: w857 -> [w884 w885]
          frame False {
          }
          frame True {
            n597 = Enqueue Element(queue=w885, element=w887) -> (queue out=w886:refnum<queue>)  [unwired: 2 in, 2 out]
          }
        }
        n598 = Enqueue Element(queue=w861, element="read current") -> (queue out=w866:refnum<queue>)  [unwired: 2 in, 2 out]
        n599 = Enqueue Element(queue=w866, element="check ramp state") -> (queue out=w860:refnum<queue>)  [unwired: 2 in, 2 out]
        n600 = case shown="True" w864 {
          tunnel: w860 -> [_ w888]
          frame False {
          }
          frame True {
            n601 = Enqueue Element(queue=w888, element="autoramp") -> ()  [unwired: 2 in, 3 out]
          }
        }
      }
      event "Auto-Ramp": Value Change {
        n602 = event-data() -> ("NewVal"=w899:bool)  [unwired: 1 in, 5 out]
        n603 = case shown="True" w899 {
          tunnel: w898 -> [_ w901]
          frame False {
          }
          frame True {
            n604 = Enqueue Element(queue=w901, element="set up autoramp times") -> ()  [unwired: 2 in, 3 out]
          }
        }
      }
      event "initialize": Value Change {
        n605 = event-data() -> ()  [unwired: 1 in, 3 out]
        n606 = local write "Ramp Magnet Up"(FALSE ("Ramp Magnet Up")) -> ()
        n607 = local write "Ramp Magnet Down"(FALSE ("Ramp Magnet Down")) -> ()
        n608 = local write "Auto-Ramp"(FALSE ("Ramp Magnet Down")) -> ()
        n609 = local read "Arduino"() -> (w905:refnum<visa-resource-name>)
        n610 = flat-sequence {
          tunnel: w905 -> [w912]
          tunnel: [w910] -> w904
          tunnel: [w909] -> w903
          tunnel: w904 -> [w915]
          tunnel: w903 -> [w914]
          tunnel: [w913] -> w902
          frame #0 {
            n611 = VISA Open(VISA resource name=w912) -> (VISA resource name=w910:refnum<visa-resource-name>, error out=w911:errorcluster)  [unwired: 4 in]
            n612 = VISA Close(VISA resource name=w910, error in (no error)=w911) -> (error out=w909:errorcluster)
          }
          frame #1 {
            n613 = VISA Clear(VISA resource name=w915, error in (no error)=w914) -> (error out=w913:errorcluster)  [unwired: 1 out]
          }
        }
        "error out" <- w902
      }
      event "Heat Switch": Value Change {
        # "Open or close the heat switch"
        n614 = event-data() -> ("NewVal"=w916:bool)  [unwired: 1 in, 5 out]
        n615 = case shown="True" w916 {
          tunnel: w917 -> [w919 w921]
          frame False {
            # "open heat switch"
            n616 = Enqueue Element(queue=w919, element="open heat switch") -> ()  [unwired: 2 in, 3 out]
          }
          frame True {
            # "close heat switch"
            n617 = Enqueue Element(queue=w921, element="close heat switch") -> ()  [unwired: 2 in, 3 out]
          }
        }
      }
      event "Ramp Magnet Up": Value Change {
        n618 = event-data() -> ("NewVal"=w922:bool)  [unwired: 1 in, 5 out]
        n619 = case shown="True" w922 {
          tunnel: w923 -> [_ w928]
          frame False {
            w925 = u16 1 items=["Ramp Up", "Soak (hold)", "Ramp Down", "Ramp up to Setpoint", "Closed Loop Feedback", "Ramp down from Setpoint", "Magnet off"] ("Ramp State")
            n620 = local write "Ramp Status"("holding" ("Ramp Status")) -> ()
            n621 = local write "Ramp State"(w925) -> ()
          }
          frame True {
            w930 = u16 2 items=["Off", "31.6 uA", "100 uA", "316 uA", "1.00 mA", "3.16 mA", "10.0 mA", "31.6 mA", "100 mA"] ("Heater Range (0: Off)")
            w931 = u16 0 items=["Ramp Up", "Ramp Down", "Ramp up to Setpoint", "Ramp down from Setpoint", "Closed Loop Feedback", "Soak (hold)"] ("Ramp State")
            n622 = local write "Ramp State"(w931) -> ()
            n623 = local write "Ramp Status"("ramping up" ("Ramp Status")) -> ()
            n624 = local write "Heater Range Set"(w930) -> ()
            n625 = Enqueue Element(queue=w928, element="open MUX relays") -> (queue out=w927:refnum<queue>)  [unwired: 2 in, 2 out]
            n626 = Enqueue Element(queue=w927, element="initialize ramp up") -> ()  [unwired: 2 in, 3 out]
          }
        }
      }
      event "Ramp Magnet Down": Value Change {
        n627 = event-data() -> ("NewVal"=w933:bool)  [unwired: 1 in, 5 out]
        n628 = case shown="True" w933 {
          tunnel: w934 -> [_ _]
          frame True {
            n629 = local read "Ramp State"() -> (w936:u16)
            n630 = case shown="0, Default" w936 {
              frame 0, Default {
                w939 = u16 2 items=["Ramp Up", "Soak (hold)", "Ramp Down", "Ramp up to Setpoint", "Closed Loop Feedback", "Ramp down from Setpoint", "Magnet off"] ("Ramp State")
                n631 = local write "Ramp State"(w939) -> ()
                n632 = local write "Ramp Magnet Up"(FALSE ("Ramp Magnet Up")) -> ()
              }
              frame 4 {
                w940 = u16 5 items=["Ramp Up", "Soak (hold)", "Ramp Down", "Ramp up to Setpoint", "Closed Loop Feedback", "Ramp down from Setpoint", "Magnet off"] ("Ramp State")
                n633 = local write "Ramp State"(w940) -> ()
              }
              frame 5 {
                w941 = u16 5 items=["Ramp Up", "Soak (hold)", "Ramp Down", "Ramp up to Setpoint", "Closed Loop Feedback", "Ramp down from Setpoint", "Magnet off"] ("Ramp State")
                n634 = local write "Ramp State"(w941) -> ()
              }
              frame 6 {
              }
            }
            n635 = local write "Ramp Status"("ramping down" ("Ramp Status")) -> ()
            n636 = local write "counter"(0.0 ("counter")) -> ()
          }
          frame False {
            w942 = u16 1 items=["Ramp Up", "Soak (hold)", "Ramp Down", "Ramp up to Setpoint", "Closed Loop Feedback", "Ramp down from Setpoint", "Magnet off"] ("Ramp State")
            n637 = local write "Ramp State"(w942) -> ()
            n638 = local write "Ramp Status"("holding" ("Ramp Status")) -> ()
          }
        }
      }
      event "Manual temp control": Value Change {
        n639 = event-data() -> ("NewVal"=w945:bool)  [unwired: 1 in, 5 out]
        n640 = case shown="False" w945 {
          tunnel: w944 -> [_ w958]
          frame False {
            w946 = u16 6 items=["Ramp Up", "Soak (hold)", "Ramp Down", "Ramp up to Setpoint", "Closed Loop Feedback", "Ramp down from Setpoint", "Magnet off"] ("Ramp State")
            w947 = u16 0 items=["Off", "31.6 uA", "100 uA", "316 uA", "1.00 mA", "3.16 mA", "10.0 mA", "31.6 mA", "100 mA"] ("Heater Range (0: Off)")
            w953 = u16 3 items=["31.6 uA", "100 uA", "316 uA", "1.00 mA", "3.16 mA", "10.0 mA", "31.6 mA", "100 mA"] ("Maximum Heater Range (0: 31.6 uA)")
            w956 = u16 3 items=["Closed Loop PID", "Zone Tuning", "Open Loop", "Off"] ("Control Mode (0: Closed Loop PID)")
            n641 = local read "ls370"() -> (w955:refnum<visa-resource-name>)
            n642 = call <instrlib>:"Config Control Mode.vi"("VISA resource name"=w955, "Control Mode (0: Closed Loop PID)"=w956, "Heater Resistance (100.00)"=10000.0, "Maximum Heater Range (0: 31.6 uA)"=w953) -> ("VISA resource name out"=w952:refnum<visa-resource-name>, "error out"=w951:errorcluster)  [unwired: 10 in]
            n643 = local read "Gain(P)"() -> (w950:dbl)
            n644 = local read "Reset(I)"() -> (w949:dbl)
            n645 = local read "Rate(D)"() -> (w948:dbl)
            n646 = call <instrlib>:"Config Control Parameters.vi"("VISA resource name"=w952, "Heater Range (0: Off)"=w947, "Gain(P) (10.000)"=w950, "Reset(I) (20)"=w949, "error in (no error)"=w951, "Rate(D) (0)"=w948) -> ()  [unwired: 8 in, 2 out]
            n647 = local write "Heater Range Set"(w947) -> ()
            n648 = local write "Ramp State"(w946) -> ()
          }
          frame True {
            # "if temp is > 500 mK, do nothing"
            n649 = local read "FAA RO600"() -> (w960:dbl)
            n650 = Less?(x=w960, y=0.5) -> (x < y?=w957:bool)
            n651 = case shown="True" w957 {
              tunnel: w958 -> [_ w964]
              frame False {
                n652 = local write "Manual temp control"(FALSE ("temp control?")) -> ()
                n653 = local write "Ramp Status"("FAA above 500 mK" ("Arduino Response 2")) -> ()
              }
              frame True {
                n654 = Enqueue Element(queue=w964, element="turn on PID feedback") -> ()  [unwired: 2 in, 3 out]
              }
            }
          }
        }
      }
      event "Calculate Autoramp Time": Value Change {
        n655 = event-data() -> ()  [unwired: 1 in, 6 out]
        n656 = Enqueue Element(queue=w966, element="Calculate ramp time") -> ()  [unwired: 2 in, 3 out]
      }
      event "Excitation Range (5: 200 uV / 100 pA)", "Autorange (0: Autorange off)", "Excitation  (T: On)": Value Change {
        n657 = event-data() -> ()  [unwired: 1 in, 6 out]
        n658 = Enqueue Element(queue=w968, element="Write LS372 Settings") -> ()  [unwired: 2 in, 3 out]
      }
      event "Query all HEMT voltages once": Value Change {
        n659 = event-data() -> ("NewVal"=w969:bool)  [unwired: 1 in, 5 out]
        n660 = case shown="True" w969 {
          tunnel: w970 -> [_ w972]
          frame False {
          }
          frame True {
            n661 = Enqueue Element(queue=w972, element="query HEMT voltages") -> ()  [unwired: 2 in, 3 out]
          }
        }
      }
      event "MUX relays": Value Change {
        n662 = event-data() -> ("NewVal"=w974:bool)  [unwired: 1 in, 5 out]
        n663 = case shown="False" w974 {
          tunnel: w973 -> [w976 w978]
          frame False {
            n664 = Enqueue Element(queue=w976, element="open MUX relays") -> ()  [unwired: 2 in, 3 out]
          }
          frame True {
            n665 = Enqueue Element(queue=w978, element="close MUX relays") -> ()  [unwired: 2 in, 3 out]
          }
        }
      }
      event "query adc magnet current once": Value Change {
        n666 = event-data() -> ()  [unwired: 1 in, 6 out]
        n667 = Enqueue Element(queue=w980, element="read adc magnet current") -> ()  [unwired: 2 in, 3 out]
      }
      event "Warmup Heater": Value Change {
        n668 = event-data() -> ("OldVal"=w983:bool)  [unwired: 1 in, 5 out]
        n669 = flat-sequence {
          tunnel: w983 -> [w985]
          tunnel: w982 -> [w984]
          tunnel: [w984] -> w981
          tunnel: w981 -> [w989]
          frame #0 {
            n670 = case shown="False" w985 {
              frame False {
                w986 = u16 0 items=["Off", "Range 1 (On)", "Range 2", "Range 3", "Range 4", "Range 5"] ("warmup heater Range")
                n671 = local write "warmup heater Range"(w986) -> ()
              }
              frame True {
                w987 = u16 1 items=["Off", "Range 1 (On)", "Range 2", "Range 3", "Range 4", "Range 5"] ("warmup heater Range")
                n672 = local write "warmup heater Range"(w987) -> ()
              }
            }
          }
          frame #1 {
            n673 = Enqueue Element(queue=w989, element="Switch Warmup Heater") -> ()  [unwired: 2 in, 3 out]
          }
        }
      }
      event "Update PID Values": Value Change {
        n674 = event-data() -> ("OldVal"=w991:bool)  [unwired: 1 in, 5 out]
        n675 = case shown="True" w991 {
          tunnel: w990 -> [_ w993]
          frame False {
          }
          frame True {
            n676 = Enqueue Element(queue=w993, element="update PID values") -> ()  [unwired: 2 in, 3 out]
          }
        }
      }
      event "Knob": Value Change {
        n677 = event-data() -> ("NewVal"=w994:i8)  [unwired: 1 in, 5 out]
        n678 = case shown="2" w994 {
          frame 0, Default {
            n679 = local read "Arduino"() -> (w995:refnum<visa-resource-name>)
            n680 = VISA Write(VISA resource name=w995, write buffer="i") -> (error out=w997:errorcluster)  [unwired: 1 in, 2 out]
            n681 = local write "error out"(w997) -> ()
          }
          frame 1 {
            n682 = local read "Arduino"() -> (w998:refnum<visa-resource-name>)
            n683 = VISA Write(VISA resource name=w998, write buffer="j") -> (error out=w1000:errorcluster)  [unwired: 1 in, 2 out]
            n684 = local write "error out"(w1000) -> ()
          }
          frame 2 {
            n685 = local read "Arduino"() -> (w1001:refnum<visa-resource-name>)
            n686 = VISA Write(VISA resource name=w1001, write buffer="k") -> (error out=w1003:errorcluster)  [unwired: 1 in, 2 out]
            n687 = local write "error out"(w1003) -> ()
          }
        }
      }
      event "Stop": Value Change {
        # "program ends here. flush queue, close connections to lakeshores"
        n688 = event-data() -> ()  [unwired: 1 in, 3 out]
        n689 = Flush Queue(queue=w1012) -> (queue out=w1007:refnum<queue>, error out=w1006:errorcluster)  [unwired: 1 in, 1 out]
        n690 = Enqueue Element At Opposite End(queue=w1007, element="False", error in (no error)=w1006) -> (queue out=w1009:refnum<queue>, error out=w1005:errorcluster)  [unwired: 1 in, 1 out]
        n691 = Enqueue Element At Opposite End(queue=w1009, element="False", error in (no error)=w1005) -> (queue out=w1004:refnum<queue>)  [unwired: 1 in, 2 out]
        n692 = local write "stopping"(TRUE ("cancelling")) -> ()
      }
    }
    n693 = local read "stopping"() -> (w845:bool)
  }
  "stopping" <- FALSE
  "GGG RO600" <- 0.0 ("1K RO600")
  "Magnet RTD" <- 0.0 ("Magnet RTD")
  "77K Diode" <- 0.0 ("4K Diode")
  "4K Diode" <- 0.0 ("77K Diode")
  "FAA RO600" <- 0.0 ("ADR RO600")
  "Sample RuOx" <- 0.0 ("Sample RuOx")
  "GGG RO600 R" <- 0.0 ("1K RO600")
  "Magnet RTD R" <- 0.0 ("Magnet RTD")
  "FAA RO600 R" <- 0.0 ("ADR RO600")
  "Sample RuOx R" <- 0.0 ("Sample RuOx")
  "Magnetic Field (kG)" <- 0.0 ("Magnet Field")
  "Ramp Status" <- "No Action" ("AutoRamp Status")
  "ramp up time (min)" <- 0.0 ("ramp up time (s)")
  "ramp down time (min)" <- 0.0 ("ramp down time (s)")
  "Arduino OK" <- FALSE ("Arduino OK")
  "counter" <- 0.0 ("x")
  "counter 2" <- 0.0 ("counter 2")
  "Reading 370" <- FALSE ("Reading 372")
  "Heater Range OK" <- FALSE ("Heater Range OK")
  "hemt v counter" <- 65 ("Numeric")
